vi "Parse Chat Reply from JSON.vi"(10 "stream":bool, 11 "Response JSON":string) -> (0 "openrouter reasoning":string, 1 "complete?":bool, 2 "message":T1, 3 "answer":string)   [LabVIEW 2023, in "LabVIEW LLM.lvlib"]
uses:
  LabVIEW LLM.lvlib
  chat-role.ctl
  chat-completion stream response.ctl
  chat-completion non-stream response.ctl
  openai_message.ctl
  <vilib>/addons/_JKI.lib/Serialization/JSON/JKI JSON Serialization.lvlib
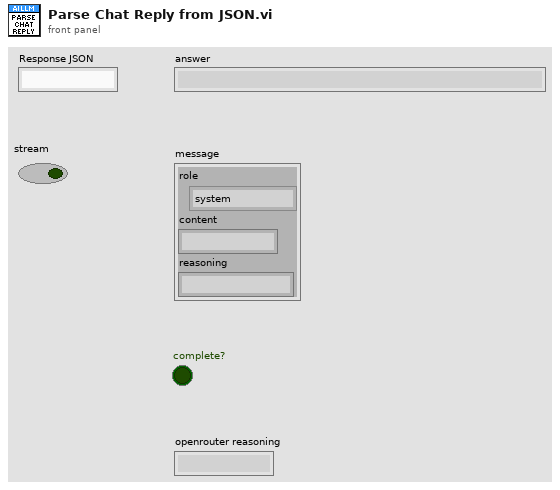
[diagram p1: front panel]
types:
  T1 = typedef "LabVIEW LLM.lvlib/openai_message.ctl" = cluster{"role":T2, "content":string, "reasoning":string}
  T2 = typedef "LabVIEW LLM.lvlib/chat-role.ctl" = enum16{"system", "user", "assistant"}
  T3 = typedef "LabVIEW LLM.lvlib/chat-completion stream response.ctl" = cluster{"id":string, "object":string, "created":i64, "model":string, "choices":cluster{"index":i64, "finish_reason":string, "delta":T1}[]}
  T4 = cluster{"index":i64, "finish_reason":string, "delta":T1}[]
  T5 = cluster{"index":i64, "finish_reason":string, "delta":T1}
  T6 = typedef "LabVIEW LLM.lvlib/chat-completion non-stream response.ctl" = cluster{"id":string, "object":string, "created":i64, "model":string, "choices":cluster{"index":i64, "finish_reason":string, "message":T1}[]}
  T7 = cluster{"index":i64, "finish_reason":string, "message":T1}[]
  T8 = cluster{"index":i64, "finish_reason":string, "message":T1}
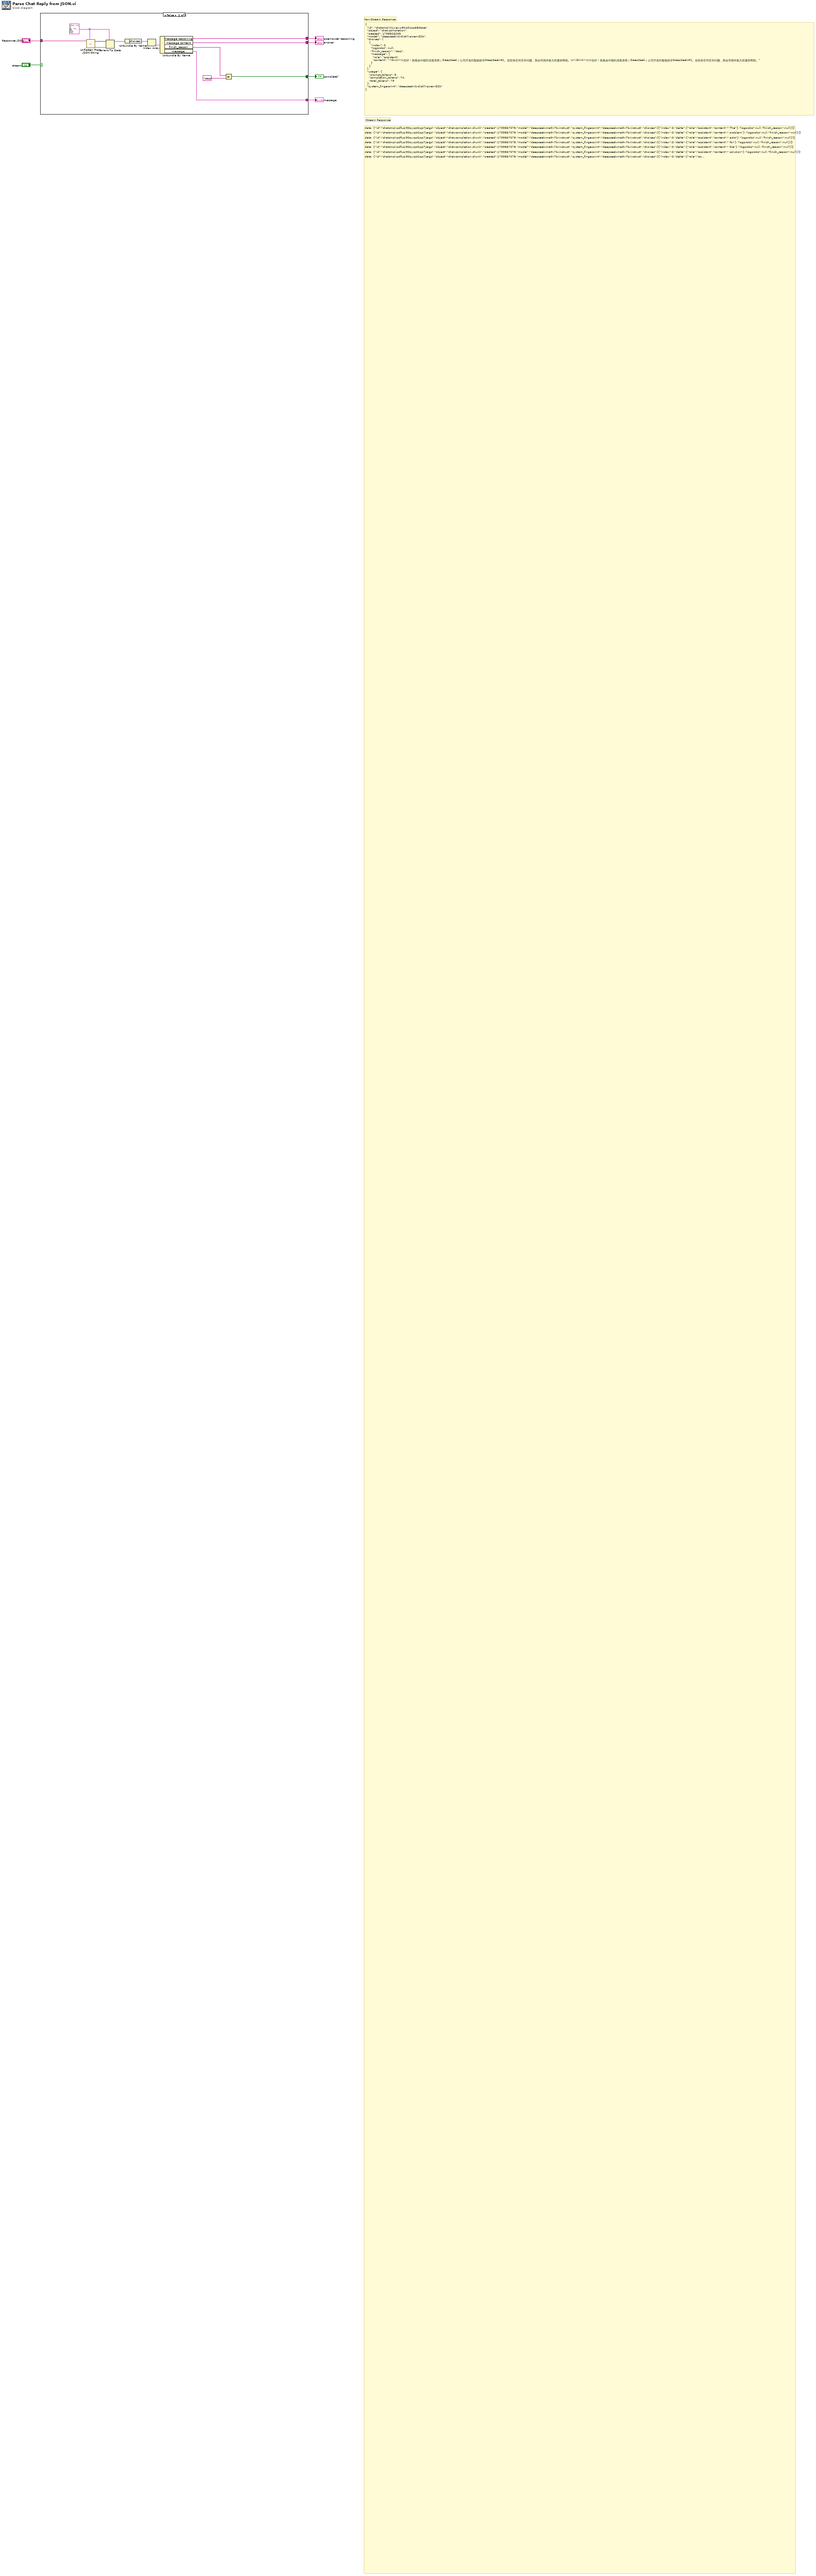
[diagram p0: block diagram]
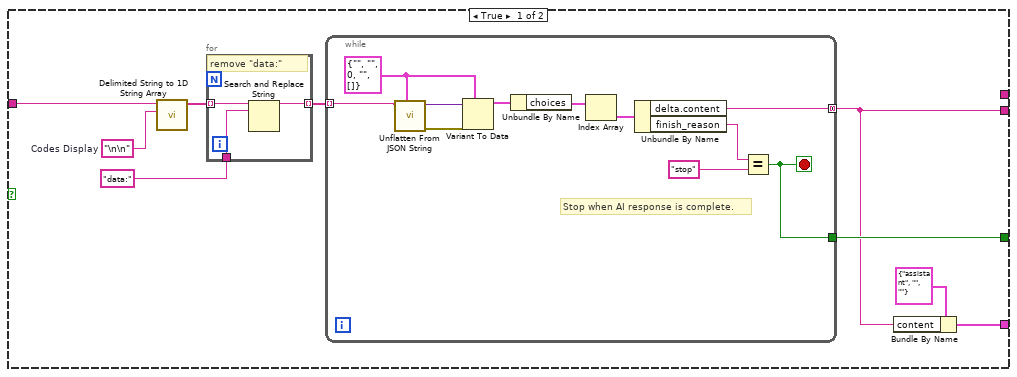
[diagram p2: hidden frame]
diagram:
  # "Non-Stream Response"
  # "Stream Response"
  # "data: {\"id\":\"chatcmpl-pdfuqi90oyqot1qp7jergc\",\"object\":\"chat.completion.chunk\",\"created\":1739867078,\"model\":\"deepseek-math-7b-instruct\",\"system_fingerprint\":\"deepseek-math-7b-instruct\",\"choices\":[{\"index\":0,\"delta\":{\"role\":\"assistant\",\"content\":\" The\"},\"logprobs\":null,\"finish_reason\":null}]}\n\ndata: {\"id\":\"chatcmpl-pdfuqi90oyqot1qp7jergc\",\"object\":\"chat.completion.chunk\",\"created\":1739867078,\"model\":\"deepseek-math-7b-instruct\",\"system_fingerprint\":\"deepseek-math-7b-instruct\",\"choices\":[{\"index\":0,\"delta\":{\"role\":\"assistant\",\"content\":\" problem\"},\"logprobs\":null,\"finish_reason\":null}]}\n\ndata: {\"id\":\"chatcmpl-pdfuqi90oyqot1qp7jergc\",\"object\":\"chat.completion.chunk\",\"created\":1739867078,\"model\":\"deepseek-math-7b-instruct\",\"system_fingerprint\":\"deepseek-math-7b-instruct\",\"choices\":[{\"index\":0,\"delta\":{\"role\":\"assistant\",\"content\":\" asks\"},\"logprobs\":null,\"finish_reason\":null}]}\n\ndata: {\"id\":\"chatcmpl-pdfuqi90oyqot1qp7jergc\",\"object\":\"chat.completion.chunk\",\"created\":1739867078,\"model\":\"deepseek-math-7b-instruct\",\"system_fingerprint\":\"deepseek-math-7b-instruct\",\"choices\":[{\"index\":0,\"delta\":{\"role\":\"assistant\",\"content\":\" for\"},\"logprobs\":null,\"finish_reason\":null}]}\n\ndata: {\"id\":\"chatcmpl-pdfuqi90oyqot1qp7jergc\",\"object\":\"chat.completion.chunk\",\"created\":1739867078,\"model\":\"deepseek-math-7b-instruct\",\"system_fingerprint\":\"deepseek-math-7b-instruct\",\"choices\":[{\"index\":0,\"delta\":{\"role\":\"assistant\",\"content\":\" the\"},\"logprobs\":null,\"finish_reason\":null}]}\n\ndata: {\"id\":\"chatcmpl-pdfuqi90oyqot1qp7jergc\",\"object\":\"chat.completion.chunk\",\"created\":1739867078,\"model\":\"deepseek-math-7b-instruct\",\"system_fingerprint\":\"deepseek-math-7b-instruct\",\"choices\":[{\"index\":0,\"delta\":{\"role\":\"assistant\",\"content\":\" solution\"},\"logprobs\":null,\"finish_reason\":null}]}\n\ndata: {\"id\":\"chatcmpl-pdfuqi90oyqot1qp7jergc\",\"object\":\"chat.completion.chunk\",\"created\":1739867078,\"model\":\"deepseek-math-7b-instruct\",\"system_fingerprint\":\"deepseek-math-7b-instruct\",\"choices\":[{\"index\":0,\"delta\":{\"role\":\"assistant\",\"content\":\" of\"},\"logprobs\":null,\"finish_reason\":null}]}\n\ndata: {\"id\":\"chatcmpl-pdfuqi90oyqot1qp7jergc\",\"object\":\"chat.completion.chunk\",\"created\":1739867078,\"model\":\"deepseek-math-7b-instruct\",\"system_fingerprint\":\"deepseek-math-7b-instruct\",\"choices\":[{\"index\":0,\"delta\":{\"role\":\"assistant\",\"content\":\"\\n\"},\"logprobs\":null,\"finish_reason\":null}]}\n\ndata: {\"id\":\"chatcmpl-pdfuqi90oyqot1qp7jergc\",\"object\":\"chat.completion.chunk\",\"created\":1739867078,\"model\":\"deepseek-math-7b-instruct\",\"system_fingerprint\":\"deepseek-math-7b-instruct\",\"choices\":[{\"index\":0,\"delta\":{\"role\":\"assistant\",\"content\":\"\\\\[\\\\\"},\"logprobs\":null,\"finish_reason\":null}]}\n\ndata: {\"id\":\"chatcmpl-pdfuqi90oyqot1qp7jergc\",\"object\":\"chat.completion.chunk\",\"created\":1739867078,\"model\":\"deepseek-math-7b-instruct\",\"system_fingerprint\":\"deepseek-math-7b-instruct\",\"choices\":[{\"index\":0,\"delta\":{\"role\":\"assistant\",\"content\":\"sin\"},\"logprobs\":null,\"finish_reason\":null}]}\n\ndata: {\"id\":\"chatcmpl-pdfuqi90oyqot1qp7jergc\",\"object\":\"chat.completion.chunk\",\"created\":1739867078,\"model\":\"deepseek-math-7b-instruct\",\"system_fingerprint\":\"deepseek-math-7b-instruct\",\"choices\":[{\"index\":0,\"delta\":{\"role\":\"assistant\",\"content\":\" x\"},\"logprobs\":null,\"finish_reason\":null}]}\n\ndata: {\"id\":\"chatcmpl-pdfuqi90oyqot1qp7jergc\",\"object\":\"chat.completion.chunk\",\"created\":1739867078,\"model\":\"deepseek-math-7b-instruct\",\"system_fingerprint\":\"deepseek-math-7b-instruct\",\"choices\":[{\"index\":0,\"delta\":{\"role\":\"assistant\",\"content\":\" +\"},\"logprobs\":null,\"finish_reason\":null}]}\n\ndata: {\"id\":\"chatcmpl-pdfuqi90oyqot1qp7jergc\",\"object\":\"chat.completion.chunk\",\"created\":1739867078,\"model\":\"deepseek-math-7b-instruct\",\"system_fingerprint\":\"deepseek-math-7b-instruct\",\"choices\":[{\"index\":0,\"delta\":{\"role\":\"assistant\",\"content\":\" \\\\\"},\"logprobs\":null,\"finish_reason\":null}]}\n\ndata: {\"id\":\"chatcmpl-pdfuqi90oyqot1qp7jergc\",\"object\":\"chat.completion.chunk\",\"created\":1739867078,\"model\":\"deepseek-math-7b-instruct\",\"system_fingerprint\":\"deepseek-math-7b-instruct\",\"choices\":[{\"index\":0,\"delta\":{\"role\":\"assistant\",\"content\":\"cos\"},\"logprobs\":null,\"finish_reason\":null}]}\n\ndata: {\"id\":\"chatcmpl-pdfuqi90oyqot1qp7jergc\",\"object\":\"chat.completion.chunk\",\"created\":1739867078,\"model\":\"deepseek-math-7b-instruct\",\"system_fingerprint\":\"deepseek-math-7b-instruct\",\"choices\":[{\"index\":0,\"delta\":{\"role\":\"assistant\",\"content\":\" \"},\"logprobs\":null,\"finish_reason\":null}]}\n\ndata: {\"id\":\"chatcmpl-pdfuqi90oyqot1qp7jergc\",\"object\":\"chat.completion.chunk\",\"created\":1739867078,\"model\":\"deepseek-math-7b-instruct\",\"system_fingerprint\":\"deepseek-math-7b-instruct\",\"choices\":[{\"index\":0,\"delta\":{\"role\":\"assistant\",\"content\":\"2\"},\"logprobs\":null,\"finish_reason\":null}]}\n\ndata: {\"id\":\"chatcmpl-pdfuqi90oyqot1qp7jergc\",\"object\":\"chat.completion.chunk\",\"created\":1739867078,\"model\":\"deepseek-math-7b-instruct\",\"system_fingerprint\":\"deepseek-math-7b-instruct\",\"choices\":[{\"index\":0,\"delta\":{\"role\":\"assistant\",\"content\":\"x\"},\"logprobs\":null,\"finish_reason\":null}]}\n\ndata: {\"id\":\"chatcmpl-pdfuqi90oyqot1qp7jergc\",\"object\":\"chat.completion.chunk\",\"created\":1739867078,\"model\":\"deepseek-math-7b-instruct\",\"system_fingerprint\":\"deepseek-math-7b-instruct\",\"choices\":[{\"index\":0,\"delta\":{\"role\":\"assistant\",\"content\":\" =\"},\"logprobs\":null,\"finish_reason\":null}]}\n\ndata: {\"id\":\"chatcmpl-pdfuqi90oyqot1qp7jergc\",\"object\":\"chat.completion.chunk\",\"created\":1739867078,\"model\":\"deepseek-math-7b-instruct\",\"system_fingerprint\":\"deepseek-math-7b-instruct\",\"choices\":[{\"index\":0,\"delta\":{\"role\":\"assistant\",\"content\":\" -\"},\"logprobs\":null,\"finish_reason\":null}]}\n\ndata: {\"id\":\"chatcmpl-pdfuqi90oyqot1qp7jergc\",\"object\":\"chat.completion.chunk\",\"created\":1739867078,\"model\":\"deepseek-math-7b-instruct\",\"system_fingerprint\":\"deepseek-math-7b-instruct\",\"choices\":[{\"index\":0,\"delta\":{\"role\":\"assistant\",\"content\":\"1\"},\"logprobs\":null,\"finish_reason\":null}]}\n\ndata: {\"id\":\"chatcmpl-pdfuqi90oyqot1qp7jergc\",\"object\":\"chat.completion.chunk\",\"created\":1739867078,\"model\":\"deepseek-math-7b-instruct\",\"system_fingerprint\":\"deepseek-math-7b-instruct\",\"choices\":[{\"index\":0,\"delta\":{\"role\":\"assistant\",\"content\":\".\\\\]\"},\"logprobs\":null,\"finish_reason\":null}]}\n\ndata: {\"id\":\"chatcmpl-pdfuqi90oyqot1qp7jergc\",\"object\":\"chat.completion.chunk\",\"created\":1739867078,\"model\":\"deepseek-math-7b-instruct\",\"system_fingerprint\":\"deepseek-math-7b-instruct\",\"choices\":[{\"index\":0,\"delta\":{\"role\":\"assistant\",\"content\":\"We\"},\"logprobs\":null,\"finish_reason\":null}]}\n\ndata: {\"id\":\"chatcmpl-pdfuqi90oyqot1qp7jergc\",\"object\":\"chat.completion.chunk\",\"created\":1739867078,\"model\":\"deepseek-math-7b-instruct\",\"system_fingerprint\":\"deepseek-math-7b-instruct\",\"choices\":[{\"index\":0,\"delta\":{\"role\":\"assistant\",\"content\":\" can\"},\"logprobs\":null,\"finish_reason\":null}]}\n\ndata: {\"id\":\"chatcmpl-pdfuqi90oyqot1qp7jergc\",\"object\":\"chat.completion.chunk\",\"created\":1739867078,\"model\":\"deepseek-math-7b-instruct\",\"system_fingerprint\":\"deepseek-math-7b-instruct\",\"choices\":[{\"index\":0,\"delta\":{\"role\":\"assistant\",\"content\":\" write\"},\"logprobs\":null,\"finish_reason\":null}]}\n\ndata: {\"id\":\"chatcmpl-pdfuqi90oyqot1qp7jergc\",\"object\":\"chat.completion.chunk\",\"created\":1739867078,\"model\":\"deepseek-math-7b-instruct\",\"system_fingerprint\":\"deepseek-math-7b-instruct\",\"choices\":[{\"index\":0,\"delta\":{\"role\":\"assistant\",\"content\":\" $\\\\\"},\"logprobs\":null,\"finish_reason\":null}]}\n\ndata: {\"id\":\"chatcmpl-pdfuqi90oyqot1qp7jergc\",\"object\":\"chat.completion.chunk\",\"created\":1739867078,\"model\":\"deepseek-math-7b-instruct\",\"system_fingerprint\":\"deepseek-math-7b-instruct\",\"choices\":[{\"index\":0,\"delta\":{\"role\":\"assistant\",\"content\":\"cos\"},\"logprobs\":null,\"finish_reason\":null}]}\n\ndata: {\"id\":\"chatcmpl-pdfuqi90oyqot1qp7jergc\",\"object\":\"chat.completion.chunk\",\"created\":1739867078,\"model\":\"deepseek-math-7b-instruct\",\"system_fingerprint\":\"deepseek-math-7b-instruct\",\"choices\":[{\"index\":0,\"delta\":{\"role\":\"assistant\",\"content\":\" \"},\"logprobs\":null,\"finish_reason\":null}]}\n\ndata: {\"id\":\"chatcmpl-pdfuqi90oyqot1qp7jergc\",\"object\":\"chat.completion.chunk\",\"created\":1739867078,\"model\":\"deepseek-math-7b-instruct\",\"system_fingerprint\":\"deepseek-math-7b-instruct\",\"choices\":[{\"index\":0,\"delta\":{\"role\":\"assistant\",\"content\":\"2\"},\"logprobs\":null,\"finish_reason\":null}]}\n\ndata: {\"id\":\"chatcmpl-pdfuqi90oyqot1qp7jergc\",\"object\":\"chat.completion.chunk\",\"created\":1739867078,\"model\":\"deepseek-math-7b-instruct\",\"system_fingerprint\":\"deepseek-math-7b-instruct\",\"choices\":[{\"index\":0,\"delta\":{\"role\":\"assistant\",\"content\":\"x\"},\"logprobs\":null,\"finish_reason\":null}]}\n\ndata: {\"id\":\"chatcmpl-pdfuqi90oyqot1qp7jergc\",\"object\":\"chat.completion.chunk\",\"created\":1739867078,\"model\":\"deepseek-math-7b-instruct\",\"system_fingerprint\":\"deepseek-math-7b-instruct\",\"choices\":[{\"index\":0,\"delta\":{\"role\":\"assistant\",\"content\":\"$\"},\"logprobs\":null,\"finish_reason\":null}]}\n\ndata: {\"id\":\"chatcmpl-pdfuqi90oyqot1qp7jergc\",\"object\":\"chat.completion.chunk\",\"created\":1739867078,\"model\":\"deepseek-math-7b-instruct\",\"system_fingerprint\":\"deepseek-math-7b-instruct\",\"choices\":[{\"index\":0,\"delta\":{\"role\":\"assistant\",\"content\":\" as\"},\"logprobs\":null,\"finish_reason\":null}]}\n\ndata: {\"id\":\"chatcmpl-pdfuqi90oyqot1qp7jergc\",\"object\":\"chat.completion.chunk\",\"created\":1739867078,\"model\":\"deepseek-math-7b-instruct\",\"system_fingerprint\":\"deepseek-math-7b-instruct\",\"choices\":[{\"index\":0,\"delta\":{\"role\":\"assistant\",\"content\":\" $\"},\"logprobs\":null,\"finish_reason\":null}]}\n\ndata: {\"id\":\"chatcmpl-pdfuqi90oyqot1qp7jergc\",\"object\":\"chat.completion.chunk\",\"created\":1739867078,\"model\":\"deepseek-math-7b-instruct\",\"system_fingerprint\":\"deepseek-math-7b-instruct\",\"choices\":[{\"index\":0,\"delta\":{\"role\":\"assistant\",\"content\":\"1\"},\"logprobs\":null,\"finish_reason\":null}]}\n\ndata: {\"id\":\"chatcmpl-pdfuqi90oyqot1qp7jergc\",\"object\":\"chat.completion.chunk\",\"created\":1739867078,\"model\":\"deepseek-math-7b-instruct\",\"system_fingerprint\":\"deepseek-math-7b-instruct\",\"choices\":[{\"index\":0,\"delta\":{\"role\":\"assistant\",\"content\":\"-\"},\"logprobs\":null,\"finish_reason\":null}]}\n\ndata: {\"id\":\"chatcmpl-pdfuqi90oyqot1qp7jergc\",\"object\":\"chat.completion.chunk\",\"created\":1739867078,\"model\":\"deepseek-math-7b-instruct\",\"system_fingerprint\":\"deepseek-math-7b-instruct\",\"choices\":[{\"index\":0,\"delta\":{\"role\":\"assistant\",\"content\":\"2\"},\"logprobs\":null,\"finish_reason\":null}]}\n\ndata: {\"id\":\"chatcmpl-pdfuqi90oyqot1qp7jergc\",\"object\":\"chat.completion.chunk\",\"created\":1739867078,\"model\":\"deepseek-math-7b-instruct\",\"system_fingerprint\":\"deepseek-math-7b-instruct\",\"choices\":[{\"index\":0,\"delta\":{\"role\":\"assistant\",\"content\":\"\\\\\"},\"logprobs\":null,\"finish_reason\":null}]}\n\ndata: {\"id\":\"chatcmpl-pdfuqi90oyqot1qp7jergc\",\"object\":\"chat.completion.chunk\",\"created\":1739867078,\"model\":\"deepseek-math-7b-instruct\",\"system_fingerprint\":\"deepseek-math-7b-instruct\",\"choices\":[{\"index\":0,\"delta\":{\"role\":\"assistant\",\"content\":\"sin\"},\"logprobs\":null,\"finish_reason\":null}]}\n\ndata: {\"id\":\"chatcmpl-pdfuqi90oyqot1qp7jergc\",\"object\":\"chat.completion.chunk\",\"created\":1739867078,\"model\":\"deepseek-math-7b-instruct\",\"system_fingerprint\":\"deepseek-math-7b-instruct\",\"choices\":[{\"index\":0,\"delta\":{\"role\":\"assistant\",\"content\":\"^\"},\"logprobs\":null,\"finish_reason\":null}]}\n\ndata: {\"id\":\"chatcmpl-pdfuqi90oyqot1qp7jergc\",\"object\":\"chat.completion.chunk\",\"created\":1739867078,\"model\":\"deepseek-math-7b-instruct\",\"system_fingerprint\":\"deepseek-math-7b-instruct\",\"choices\":[{\"index\":0,\"delta\":{\"role\":\"assistant\",\"content\":\"2\"},\"logprobs\":null,\"finish_reason\":null}]}\n\ndata: {\"id\":\"chatcmpl-pdfuqi90oyqot1qp7jergc\",\"object\":\"chat.completion.chunk\",\"created\":1739867078,\"model\":\"deepseek-math-7b-instruct\",\"system_fingerprint\":\"deepseek-math-7b-instruct\",\"choices\":[{\"index\":0,\"delta\":{\"role\":\"assistant\",\"content\":\" x\"},\"logprobs\":null,\"finish_reason\":null}]}\n\ndata: {\"id\":\"chatcmpl-pdfuqi90oyqot1qp7jergc\",\"object\":\"chat.completion.chunk\",\"created\":1739867078,\"model\":\"deepseek-math-7b-instruct\",\"system_fingerprint\":\"deepseek-math-7b-instruct\",\"choices\":[{\"index\":0,\"delta\":{\"role\":\"assistant\",\"content\":\"$,\"},\"logprobs\":null,\"finish_reason\":null}]}\n\ndata: {\"id\":\"chatcmpl-pdfuqi90oyqot1qp7jergc\",\"object\":\"chat.completion.chunk\",\"created\":1739867078,\"model\":\"deepseek-math-7b-instruct\",\"system_fingerprint\":\"deepseek-math-7b-instruct\",\"choices\":[{\"index\":0,\"delta\":{\"role\":\"assistant\",\"content\":\" so\"},\"logprobs\":null,\"finish_reason\":null}]}\n\ndata: {\"id\":\"chatcmpl-pdfuqi90oyqot1qp7jergc\",\"object\":\"chat.completion.chunk\",\"created\":1739867078,\"model\":\"deepseek-math-7b-instruct\",\"system_fingerprint\":\"deepseek-math-7b-instruct\",\"choices\":[{\"index\":0,\"delta\":{\"role\":\"assistant\",\"content\":\" we\"},\"logprobs\":null,\"finish_reason\":null}]}\n\ndata: {\"id\":\"chatcmpl-pdfuqi90oyqot1qp7jergc\",\"object\":\"chat.completion.chunk\",\"created\":1739867078,\"model\":\"deepseek-math-7b-instruct\",\"system_fingerprint\":\"deepseek-math-7b-instruct\",\"choices\":[{\"index\":0,\"delta\":{\"role\":\"assistant\",\"content\":\" have\"},\"logprobs\":null,\"finish_reason\":null}]}\n\ndata: {\"id\":\"chatcmpl-pdfuqi90oyqot1qp7jergc\",\"object\":\"chat.completion.chunk\",\"created\":1739867078,\"model\":\"deepseek-math-7b-instruct\",\"system_fingerprint\":\"deepseek-math-7b-instruct\",\"choices\":[{\"index\":0,\"delta\":{\"role\":\"assistant\",\"content\":\" \\\\[\\\\\"},\"logprobs\":null,\"finish_reason\":null}]}\n\ndata: {\"id\":\"chatcmpl-pdfuqi90oyqot1qp7jergc\",\"object\":\"chat.completion.chunk\",\"created\":1739867078,\"model\":\"deepseek-math-7b-instruct\",\"system_fingerprint\":\"deepseek-math-7b-instruct\",\"choices\":[{\"index\":0,\"delta\":{\"role\":\"assistant\",\"content\":\"sin\"},\"logprobs\":null,\"finish_reason\":null}]}\n\ndata: {\"id\":\"chatcmpl-pdfuqi90oyqot1qp7jergc\",\"object\":\"chat.completion.chunk\",\"created\":1739867078,\"model\":\"deepseek-math-7b-instruct\",\"system_fingerprint\":\"deepseek-math-7b-instruct\",\"choices\":[{\"index\":0,\"delta\":{\"role\":\"assistant\",\"content\":\" x\"},\"logprobs\":null,\"finish_reason\":null}]}\n\ndata: {\"id\":\"chatcmpl-pdfuqi90oyqot1qp7jergc\",\"object\":\"chat.completion.chunk\",\"created\":1739867078,\"model\":\"deepseek-math-7b-instruct\",\"system_fingerprint\":\"deepseek-math-7b-instruct\",\"choices\":[{\"index\":0,\"delta\":{\"role\":\"assistant\",\"content\":\" +\"},\"logprobs\":null,\"finish_reason\":null}]}\n\ndata: {\"id\":\"chatcmpl-pdfuqi90oyqot1qp7jergc\",\"object\":\"chat.completion.chunk\",\"created\":1739867078,\"model\":\"deepseek-math-7b-instruct\",\"system_fingerprint\":\"deepseek-math-7b-instruct\",\"choices\":[{\"index\":0,\"delta\":{\"role\":\"assistant\",\"content\":\" (\"},\"logprobs\":null,\"finish_reason\":null}]}\n\ndata: {\"id\":\"chatcmpl-pdfuqi90oyqot1qp7jergc\",\"object\":\"chat.completion.chunk\",\"created\":1739867078,\"model\":\"deepseek-math-7b-instruct\",\"system_fingerprint\":\"deepseek-math-7b-instruct\",\"choices\":[{\"index\":0,\"delta\":{\"role\":\"assistant\",\"content\":\"1\"},\"logprobs\":null,\"finish_reason\":null}]}\n\ndata: {\"id\":\"chatcmpl-pdfuqi90oyqot1qp7jergc\",\"object\":\"chat.completion.chunk\",\"created\":1739867078,\"model\":\"deepseek-math-7b-instruct\",\"system_fingerprint\":\"deepseek-math-7b-instruct\",\"choices\":[{\"index\":0,\"delta\":{\"role\":\"assistant\",\"content\":\" -\"},\"logprobs\":null,\"finish_reason\":null}]}\n\ndata: {\"id\":\"chatcmpl-pdfuqi90oyqot1qp7jergc\",\"object\":\"chat.completion.chunk\",\"created\":1739867078,\"model\":\"deepseek-math-7b-instruct\",\"system_fingerprint\":\"deepseek-math-7b-instruct\",\"choices\":[{\"index\":0,\"delta\":{\"role\":\"assistant\",\"content\":\" \"},\"logprobs\":null,\"finish_reason\":null}]}\n\ndata: {\"id\":\"chatcmpl-pdfuqi90oyqot1qp7jergc\",\"object\":\"chat.completion.chunk\",\"created\":1739867078,\"model\":\"deepseek-math-7b-instruct\",\"system_fingerprint\":\"deepseek-math-7b-instruct\",\"choices\":[{\"index\":0,\"delta\":{\"role\":\"assistant\",\"content\":\"2\"},\"logprobs\":null,\"finish_reason\":null}]}\n\ndata: {\"id\":\"chatcmpl-pdfuqi90oyqot1qp7jergc\",\"object\":\"chat.completion.chunk\",\"created\":1739867078,\"model\":\"deepseek-math-7b-instruct\",\"system_fingerprint\":\"deepseek-math-7b-instruct\",\"choices\":[{\"index\":0,\"delta\":{\"role\":\"assistant\",\"content\":\"\\\\\"},\"logprobs\":null,\"finish_reason\":null}]}\n\ndata: {\"id\":\"chatcmpl-pdfuqi90oyqot1qp7jergc\",\"object\":\"chat.completion.chunk\",\"created\":1739867078,\"model\":\"deepseek-math-7b-instruct\",\"system_fingerprint\":\"deepseek-math-7b-instruct\",\"choices\":[{\"index\":0,\"delta\":{\"role\":\"assistant\",\"content\":\"sin\"},\"logprobs\":null,\"finish_reason\":null}]}\n\ndata: {\"id\":\"chatcmpl-pdfuqi90oyqot1qp7jergc\",\"object\":\"chat.completion.chunk\",\"created\":1739867078,\"model\":\"deepseek-math-7b-instruct\",\"system_fingerprint\":\"deepseek-math-7b-instruct\",\"choices\":[{\"index\":0,\"delta\":{\"role\":\"assistant\",\"content\":\"^\"},\"logprobs\":null,\"finish_reason\":null}]}\n\ndata: {\"id\":\"chatcmpl-pdfuqi90oyqot1qp7jergc\",\"object\":\"chat.completion.chunk\",\"created\":1739867078,\"model\":\"deepseek-math-7b-instruct\",\"system_fingerprint\":\"deepseek-math-7b-instruct\",\"choices\":[{\"index\":0,\"delta\":{\"role\":\"assistant\",\"content\":\"2\"},\"logprobs\":null,\"finish_reason\":null}]}\n\ndata: {\"id\":\"chatcmpl-pdfuqi90oyqot1qp7jergc\",\"object\":\"chat.completion.chunk\",\"created\":1739867078,\"model\":\"deepseek-math-7b-instruct\",\"system_fingerprint\":\"deepseek-math-7b-instruct\",\"choices\":[{\"index\":0,\"delta\":{\"role\":\"assistant\",\"content\":\" x\"},\"logprobs\":null,\"finish_reason\":null}]}\n\ndata: {\"id\":\"chatcmpl-pdfuqi90oyqot1qp7jergc\",\"object\":\"chat.completion.chunk\",\"created\":1739867078,\"model\":\"deepseek-math-7b-instruct\",\"system_fingerprint\":\"deepseek-math-7b-instruct\",\"choices\":[{\"index\":0,\"delta\":{\"role\":\"assistant\",\"content\":\")\"},\"logprobs\":null,\"finish_reason\":null}]}\n\ndata: {\"id\":\"chatcmpl-pdfuqi90oyqot1qp7jergc\",\"object\":\"chat.completion.chunk\",\"created\":1739867078,\"model\":\"deepseek-math-7b-instruct\",\"system_fingerprint\":\"deepseek-math-7b-instruct\",\"choices\":[{\"index\":0,\"delta\":{\"role\":\"assistant\",\"content\":\" =\"},\"logprobs\":null,\"finish_reason\":null}]}\n\ndata: {\"id\":\"chatcmpl-pdfuqi90oyqot1qp7jergc\",\"object\":\"chat.completion.chunk\",\"created\":1739867078,\"model\":\"deepseek-math-7b-instruct\",\"system_fingerprint\":\"deepseek-math-7b-instruct\",\"choices\":[{\"index\":0,\"delta\":{\"role\":\"assistant\",\"content\":\" -\"},\"logprobs\":null,\"finish_reason\":null}]}\n\ndata: {\"id\":\"chatcmpl-pdfuqi90oyqot1qp7jergc\",\"object\":\"chat.completion.chunk\",\"created\":1739867078,\"model\":\"deepseek-math-7b-instruct\",\"system_fingerprint\":\"deepseek-math-7b-instruct\",\"choices\":[{\"index\":0,\"delta\":{\"role\":\"assistant\",\"content\":\"1\"},\"logprobs\":null,\"finish_reason\":null}]}\n\ndata: {\"id\":\"chatcmpl-pdfuqi90oyqot1qp7jergc\",\"object\":\"chat.completion.chunk\",\"created\":1739867078,\"model\":\"deepseek-math-7b-instruct\",\"system_fingerprint\":\"deepseek-math-7b-instruct\",\"choices\":[{\"index\":0,\"delta\":{\"role\":\"assistant\",\"content\":\",\\\\]\"},\"logprobs\":null,\"finish_reason\":null}]}\n\ndata: {\"id\":\"chatcmpl-pdfuqi90oyqot1qp7jergc\",\"object\":\"chat.completion.chunk\",\"created\":1739867078,\"model\":\"deepseek-math-7b-instruct\",\"system_fingerprint\":\"deepseek-math-7b-instruct\",\"choices\":[{\"index\":0,\"delta\":{\"role\":\"assistant\",\"content\":\"which\"},\"logprobs\":null,\"finish_reason\":null}]}\n\ndata: {\"id\":\"chatcmpl-pdfuqi90oyqot1qp7jergc\",\"object\":\"chat.completion.chunk\",\"created\":1739867078,\"model\":\"deepseek-math-7b-instruct\",\"system_fingerprint\":\"deepseek-math-7b-instruct\",\"choices\":[{\"index\":0,\"delta\":{\"role\":\"assistant\",\"content\":\" simplifies\"},\"logprobs\":null,\"finish_reason\":null}]}\n\ndata: {\"id\":\"chatcmpl-pdfuqi90oyqot1qp7jergc\",\"object\":\"chat.completion.chunk\",\"created\":1739867078,\"model\":\"deepseek-math-7b-instruct\",\"system_fingerprint\":\"deepseek-math-7b-instruct\",\"choices\":[{\"index\":0,\"delta\":{\"role\":\"assistant\",\"content\":\" to\"},\"logprobs\":null,\"finish_reason\":null}]}\n\ndata: {\"id\":\"chatcmpl-pdfuqi90oyqot1qp7jergc\",\"object\":\"chat.completion.chunk\",\"created\":1739867078,\"model\":\"deepseek-math-7b-instruct\",\"system_fingerprint\":\"deepseek-math-7b-instruct\",\"choices\":[{\"index\":0,\"delta\":{\"role\":\"assistant\",\"content\":\" \\\\[\"},\"logprobs\":null,\"finish_reason\":null}]}\n\ndata: {\"id\":\"chatcmpl-pdfuqi90oyqot1qp7jergc\",\"object\":\"chat.completion.chunk\",\"created\":1739867078,\"model\":\"deepseek-math-7b-instruct\",\"system_fingerprint\":\"deepseek-math-7b-instruct\",\"choices\":[{\"index\":0,\"delta\":{\"role\":\"assistant\",\"content\":\"0\"},\"logprobs\":null,\"finish_reason\":null}]}\n\ndata: {\"id\":\"chatcmpl-pdfuqi90oyqot1qp7jergc\",\"object\":\"chat.completion.chunk\",\"created\":1739867078,\"model\":\"deepseek-math-7b-instruct\",\"system_fingerprint\":\"deepseek-math-7b-instruct\",\"choices\":[{\"index\":0,\"delta\":{\"role\":\"assistant\",\"content\":\"=\"},\"logprobs\":null,\"finish_reason\":null}]}\n\ndata: {\"id\":\"chatcmpl-pdfuqi90oyqot1qp7jergc\",\"object\":\"chat.completion.chunk\",\"created\":1739867078,\"model\":\"deepseek-math-7b-instruct\",\"system_fingerprint\":\"deepseek-math-7b-instruct\",\"choices\":[{\"index\":0,\"delta\":{\"role\":\"assistant\",\"content\":\"2\"},\"logprobs\":null,\"finish_reason\":null}]}\n\ndata: {\"id\":\"chatcmpl-pdfuqi90oyqot1qp7jergc\",\"object\":\"chat.completion.chunk\",\"created\":1739867078,\"model\":\"deepseek-math-7b-instruct\",\"system_fingerprint\":\"deepseek-math-7b-instruct\",\"choices\":[{\"index\":0,\"delta\":{\"role\":\"assistant\",\"content\":\"\\\\\"},\"logprobs\":null,\"finish_reason\":null}]}\n\ndata: {\"id\":\"chatcmpl-pdfuqi90oyqot1qp7jergc\",\"object\":\"chat.completion.chunk\",\"created\":1739867078,\"model\":\"deepseek-math-7b-instruct\",\"system_fingerprint\":\"deepseek-math-7b-instruct\",\"choices\":[{\"index\":0,\"delta\":{\"role\":\"assistant\",\"content\":\"sin\"},\"logprobs\":null,\"finish_reason\":null}]}\n\ndata: {\"id\":\"chatcmpl-pdfuqi90oyqot1qp7jergc\",\"object\":\"chat.completion.chunk\",\"created\":1739867078,\"model\":\"deepseek-math-7b-instruct\",\"system_fingerprint\":\"deepseek-math-7b-instruct\",\"choices\":[{\"index\":0,\"delta\":{\"role\":\"assistant\",\"content\":\" ^\"},\"logprobs\":null,\"finish_reason\":null}]}\n\ndata: {\"id\":\"chatcmpl-pdfuqi90oyqot1qp7jergc\",\"object\":\"chat.completion.chunk\",\"created\":1739867078,\"model\":\"deepseek-math-7b-instruct\",\"system_fingerprint\":\"deepseek-math-7b-instruct\",\"choices\":[{\"index\":0,\"delta\":{\"role\":\"assistant\",\"content\":\"2\"},\"logprobs\":null,\"finish_reason\":null}]}\n\ndata: {\"id\":\"chatcmpl-pdfuqi90oyqot1qp7jergc\",\"object\":\"chat.completion.chunk\",\"created\":1739867078,\"model\":\"deepseek-math-7b-instruct\",\"system_fingerprint\":\"deepseek-math-7b-instruct\",\"choices\":[{\"index\":0,\"delta\":{\"role\":\"assistant\",\"content\":\"(\"},\"logprobs\":null,\"finish_reason\":null}]}\n\ndata: {\"id\":\"chatcmpl-pdfuqi90oyqot1qp7jergc\",\"object\":\"chat.completion.chunk\",\"created\":1739867078,\"model\":\"deepseek-math-7b-instruct\",\"system_fingerprint\":\"deepseek-math-7b-instruct\",\"choices\":[{\"index\":0,\"delta\":{\"role\":\"assistant\",\"content\":\"x\"},\"logprobs\":null,\"finish_reason\":null}]}\n\ndata: {\"id\":\"chatcmpl-pdfuqi90oyqot1qp7jergc\",\"object\":\"chat.completion.chunk\",\"created\":1739867078,\"model\":\"deepseek-math-7b-instruct\",\"system_fingerprint\":\"deepseek-math-7b-instruct\",\"choices\":[{\"index\":0,\"delta\":{\"role\":\"assistant\",\"content\":\")+\\\\\"},\"logprobs\":null,\"finish_reason\":null}]}\n\ndata: {\"id\":\"chatcmpl-pdfuqi90oyqot1qp7jergc\",\"object\":\"chat.completion.chunk\",\"created\":1739867078,\"model\":\"deepseek-math-7b-instruct\",\"system_fingerprint\":\"deepseek-math-7b-instruct\",\"choices\":[{\"index\":0,\"delta\":{\"role\":\"assistant\",\"content\":\"sin\"},\"logprobs\":null,\"finish_reason\":null}]}\n\ndata: {\"id\":\"chatcmpl-pdfuqi90oyqot1qp7jergc\",\"object\":\"chat.completion.chunk\",\"created\":1739867078,\"model\":\"deepseek-math-7b-instruct\",\"system_fingerprint\":\"deepseek-math-7b-instruct\",\"choices\":[{\"index\":0,\"delta\":{\"role\":\"assistant\",\"content\":\"(\"},\"logprobs\":null,\"finish_reason\":null}]}\n\ndata: {\"id\":\"chatcmpl-pdfuqi90oyqot1qp7jergc\",\"object\":\"chat.completion.chunk\",\"created\":1739867078,\"model\":\"deepseek-math-7b-instruct\",\"system_fingerprint\":\"deepseek-math-7b-instruct\",\"choices\":[{\"index\":0,\"delta\":{\"role\":\"assistant\",\"content\":\"x\"},\"logprobs\":null,\"finish_reason\":null}]}\n\ndata: {\"id\":\"chatcmpl-pdfuqi90oyqot1qp7jergc\",\"object\":\"chat.completion.chunk\",\"created\":1739867078,\"model\":\"deepseek-math-7b-instruct\",\"system_fingerprint\":\"deepseek-math-7b-instruct\",\"choices\":[{\"index\":0,\"delta\":{\"role\":\"assistant\",\"content\":\")+\"},\"logprobs\":null,\"finish_reason\":null}]}\n\ndata: {\"id\":\"chatcmpl-pdfuqi90oyqot1qp7jergc\",\"object\":\"chat.completion.chunk\",\"created\":1739867078,\"model\":\"deepseek-math-7b-instruct\",\"system_fingerprint\":\"deepseek-math-7b-instruct\",\"choices\":[{\"index\":0,\"delta\":{\"role\":\"assistant\",\"content\":\"1\"},\"logprobs\":null,\"finish_reason\":null}]}\n\ndata: {\"id\":\"chatcmpl-pdfuqi90oyqot1qp7jergc\",\"object\":\"chat.completion.chunk\",\"created\":1739867078,\"model\":\"deepseek-math-7b-instruct\",\"system_fingerprint\":\"deepseek-math-7b-instruct\",\"choices\":[{\"index\":0,\"delta\":{\"role\":\"assistant\",\"content\":\"\\\\]\"},\"logprobs\":null,\"finish_reason\":null}]}\n\ndata: {\"id\":\"chatcmpl-pdfuqi90oyqot1qp7jergc\",\"object\":\"chat.completion.chunk\",\"created\":1739867078,\"model\":\"deepseek-math-7b-instruct\",\"system_fingerprint\":\"deepseek-math-7b-instruct\",\"choices\":[{\"index\":0,\"delta\":{\"role\":\"assistant\",\"content\":\"or\"},\"logprobs\":null,\"finish_reason\":null}]}\n\ndata: {\"id\":\"chatcmpl-pdfuqi90oyqot1qp7jergc\",\"object\":\"chat.completion.chunk\",\"created\":1739867078,\"model\":\"deepseek-math-7b-instruct\",\"system_fingerprint\":\"deepseek-math-7b-instruct\",\"choices\":[{\"index\":0,\"delta\":{\"role\":\"assistant\",\"content\":\",\"},\"logprobs\":null,\"finish_reason\":null}]}\n\ndata: {\"id\":\"chatcmpl-pdfuqi90oyqot1qp7jergc\",\"object\":\"chat.completion.chunk\",\"created\":1739867078,\"model\":\"deepseek-math-7b-instruct\",\"system_fingerprint\":\"deepseek-math-7b-instruct\",\"choices\":[{\"index\":0,\"delta\":{\"role\":\"assistant\",\"content\":\" equivalently\"},\"logprobs\":null,\"finish_reason\":null}]}\n\ndata: {\"id\":\"chatcmpl-pdfuqi90oyqot1qp7jergc\",\"object\":\"chat.completion.chunk\",\"created\":1739867078,\"model\":\"deepseek-math-7b-instruct\",\"system_fingerprint\":\"deepseek-math-7b-instruct\",\"choices\":[{\"index\":0,\"delta\":{\"role\":\"assistant\",\"content\":\",\\\\\"},\"logprobs\":null,\"finish_reason\":null}]}\n\ndata: {\"id\":\"chatcmpl-pdfuqi90oyqot1qp7jergc\",\"object\":\"chat.completion.chunk\",\"created\":1739867078,\"model\":\"deepseek-math-7b-instruct\",\"system_fingerprint\":\"deepseek-math-7b-instruct\",\"choices\":[{\"index\":0,\"delta\":{\"role\":\"assistant\",\"content\":\"[\"},\"logprobs\":null,\"finish_reason\":null}]}\n\ndata: {\"id\":\"chatcmpl-pdfuqi90oyqot1qp7jergc\",\"object\":\"chat.completion.chunk\",\"created\":1739867078,\"model\":\"deepseek-math-7b-instruct\",\"system_fingerprint\":\"deepseek-math-7b-instruct\",\"choices\":[{\"index\":0,\"delta\":{\"role\":\"assistant\",\"content\":\"2\"},\"logprobs\":null,\"finish_reason\":null}]}\n\ndata: {\"id\":\"chatcmpl-pdfuqi90oyqot1qp7jergc\",\"object\":\"chat.completion.chunk\",\"created\":1739867078,\"model\":\"deepseek-math-7b-instruct\",\"system_fingerprint\":\"deepseek-math-7b-instruct\",\"choices\":[{\"index\":0,\"delta\":{\"role\":\"assistant\",\"content\":\" \\\\\"},\"logprobs\":null,\"finish_reason\":null}]}\n\ndata: {\"id\":\"chatcmpl-pdfuqi90oyqot1qp7jergc\",\"object\":\"chat.completion.chunk\",\"created\":1739867078,\"model\":\"deepseek-math-7b-instruct\",\"system_fingerprint\":\"deepseek-math-7b-instruct\",\"choices\":[{\"index\":0,\"delta\":{\"role\":\"assistant\",\"content\":\"sin\"},\"logprobs\":null,\"finish_reason\":null}]}\n\ndata: {\"id\":\"chatcmpl-pdfuqi90oyqot1qp7jergc\",\"object\":\"chat.completion.chunk\",\"created\":1739867078,\"model\":\"deepseek-math-7b-instruct\",\"system_fingerprint\":\"deepseek-math-7b-instruct\",\"choices\":[{\"index\":0,\"delta\":{\"role\":\"assistant\",\"content\":\"^\"},\"logprobs\":null,\"finish_reason\":null}]}\n\ndata: {\"id\":\"chatcmpl-pdfuqi90oyqot1qp7jergc\",\"object\":\"chat.completion.chunk\",\"created\":1739867078,\"model\":\"deepseek-math-7b-instruct\",\"system_fingerprint\":\"deepseek-math-7b-instruct\",\"choices\":[{\"index\":0,\"delta\":{\"role\":\"assistant\",\"content\":\"2\"},\"logprobs\":null,\"finish_reason\":null}]}\n\ndata: {\"id\":\"chatcmpl-pdfuqi90oyqot1qp7jergc\",\"object\":\"chat.completion.chunk\",\"created\":1739867078,\"model\":\"deepseek-math-7b-instruct\",\"system_fingerprint\":\"deepseek-math-7b-instruct\",\"choices\":[{\"index\":0,\"delta\":{\"role\":\"assistant\",\"content\":\" x\"},\"logprobs\":null,\"finish_reason\":null}]}\n\ndata: {\"id\":\"chatcmpl-pdfuqi90oyqot1qp7jergc\",\"object\":\"chat.completion.chunk\",\"created\":1739867078,\"model\":\"deepseek-math-7b-instruct\",\"system_fingerprint\":\"deepseek-math-7b-instruct\",\"choices\":[{\"index\":0,\"delta\":{\"role\":\"assistant\",\"content\":\"+\\\\\"},\"logprobs\":null,\"finish_reason\":null}]}\n\ndata: {\"id\":\"chatcmpl-pdfuqi90oyqot1qp7jergc\",\"object\":\"chat.completion.chunk\",\"created\":1739867078,\"model\":\"deepseek-math-7b-instruct\",\"system_fingerprint\":\"deepseek-math-7b-instruct\",\"choices\":[{\"index\":0,\"delta\":{\"role\":\"assistant\",\"content\":\"sin\"},\"logprobs\":null,\"finish_reason\":null}]}\n\ndata: {\"id\":\"chatcmpl-pdfuqi90oyqot1qp7jergc\",\"object\":\"chat.completion.chunk\",\"created\":1739867078,\"model\":\"deepseek-math-7b-instruct\",\"system_fingerprint\":\"deepseek-math-7b-instruct\",\"choices\":[{\"index\":0,\"delta\":{\"role\":\"assistant\",\"content\":\" x\"},\"logprobs\":null,\"finish_reason\":null}]}\n\ndata: {\"id\":\"chatcmpl-pdfuqi90oyqot1qp7jergc\",\"object\":\"chat.completion.chunk\",\"created\":1739867078,\"model\":\"deepseek-math-7b-instruct\",\"system_fingerprint\":\"deepseek-math-7b-instruct\",\"choices\":[{\"index\":0,\"delta\":{\"role\":\"assistant\",\"content\":\"+\"},\"logprobs\":null,\"finish_reason\":null}]}\n\ndata: {\"id\":\"chatcmpl-pdfuqi90oyqot1qp7jergc\",\"object\":\"chat.completion.chunk\",\"created\":1739867078,\"model\":\"deepseek-math-7b-instruct\",\"system_fingerprint\":\"deepseek-math-7b-instruct\",\"choices\":[{\"index\":0,\"delta\":{\"role\":\"assistant\",\"content\":\"1\"},\"logprobs\":null,\"finish_reason\":null}]}\n\ndata: {\"id\":\"chatcmpl-pdfuqi90oyqot1qp7jergc\",\"object\":\"chat.completion.chunk\",\"created\":1739867078,\"model\":\"deepseek-math-7b-instruct\",\"system_fingerprint\":\"deepseek-math-7b-instruct\",\"choices\":[{\"index\":0,\"delta\":{\"role\":\"assistant\",\"content\":\"=(\"},\"logprobs\":null,\"finish_reason\":null}]}\n\ndata: {\"id\":\"chatcmpl-pdfuqi90oyqot1qp7jergc\",\"object\":\"chat.completion.chunk\",\"created\":1739867078,\"model\":\"deepseek-math-7b-instruct\",\"system_fingerprint\":\"deepseek-math-7b-instruct\",\"choices\":[{\"index\":0,\"delta\":{\"role\":\"assistant\",\"content\":\"2\"},\"logprobs\":null,\"finish_reason\":null}]}\n\ndata: {\"id\":\"chatcmpl-pdfuqi90oyqot1qp7jergc\",\"object\":\"chat.completion.chunk\",\"created\":1739867078,\"model\":\"deepseek-math-7b-instruct\",\"system_fingerprint\":\"deepseek-math-7b-instruct\",\"choices\":[{\"index\":0,\"delta\":{\"role\":\"assistant\",\"content\":\" \\\\\"},\"logprobs\":null,\"finish_reason\":null}]}\n\ndata: {\"id\":\"chatcmpl-pdfuqi90oyqot1qp7jergc\",\"object\":\"chat.completion.chunk\",\"created\":1739867078,\"model\":\"deepseek-math-7b-instruct\",\"system_fingerprint\":\"deepseek-math-7b-instruct\",\"choices\":[{\"index\":0,\"delta\":{\"role\":\"assistant\",\"content\":\"sin\"},\"logprobs\":null,\"finish_reason\":null}]}\n\ndata: {\"id\":\"chatcmpl-pdfuqi90oyqot1qp7jergc\",\"object\":\"chat.completion.chunk\",\"created\":1739867078,\"model\":\"deepseek-math-7b-instruct\",\"system_fingerprint\":\"deepseek-math-7b-instruct\",\"choices\":[{\"index\":0,\"delta\":{\"role\":\"assistant\",\"content\":\" x\"},\"logprobs\":null,\"finish_reason\":null}]}\n\ndata: {\"id\":\"chatcmpl-pdfuqi90oyqot1qp7jergc\",\"object\":\"chat.completion.chunk\",\"created\":1739867078,\"model\":\"deepseek-math-7b-instruct\",\"system_fingerprint\":\"deepseek-math-7b-instruct\",\"choices\":[{\"index\":0,\"delta\":{\"role\":\"assistant\",\"content\":\"+\"},\"logprobs\":null,\"finish_reason\":null}]}\n\ndata: {\"id\":\"chatcmpl-pdfuqi90oyqot1qp7jergc\",\"object\":\"chat.completion.chunk\",\"created\":1739867078,\"model\":\"deepseek-math-7b-instruct\",\"system_fingerprint\":\"deepseek-math-7b-instruct\",\"choices\":[{\"index\":0,\"delta\":{\"role\":\"assistant\",\"content\":\"1\"},\"logprobs\":null,\"finish_reason\":null}]}\n\ndata: {\"id\":\"chatcmpl-pdfuqi90oyqot1qp7jergc\",\"object\":\"chat.completion.chunk\",\"created\":1739867078,\"model\":\"deepseek-math-7b-instruct\",\"system_fingerprint\":\"deepseek-math-7b-instruct\",\"choices\":[{\"index\":0,\"delta\":{\"role\":\"assistant\",\"content\":\")(\\\\\"},\"logprobs\":null,\"finish_reason\":null}]}\n\ndata: {\"id\":\"chatcmpl-pdfuqi90oyqot1qp7jergc\",\"object\":\"chat.completion.chunk\",\"created\":1739867078,\"model\":\"deepseek-math-7b-instruct\",\"system_fingerprint\":\"deepseek-math-7b-instruct\",\"choices\":[{\"index\":0,\"delta\":{\"role\":\"assistant\",\"content\":\"sin\"},\"logprobs\":null,\"finish_reason\":null}]}\n\ndata: {\"id\":\"chatcmpl-pdfuqi90oyqot1qp7jergc\",\"object\":\"chat.completion.chunk\",\"created\":1739867078,\"model\":\"deepseek-math-7b-instruct\",\"system_fingerprint\":\"deepseek-math-7b-instruct\",\"choices\":[{\"index\":0,\"delta\":{\"role\":\"assistant\",\"content\":\" x\"},\"logprobs\":null,\"finish_reason\":null}]}\n\ndata: {\"id\":\"chatcmpl-pdfuqi90oyqot1qp7jergc\",\"object\":\"chat.completion.chunk\",\"created\":1739867078,\"model\":\"deepseek-math-7b-instruct\",\"system_fingerprint\":\"deepseek-math-7b-instruct\",\"choices\":[{\"index\":0,\"delta\":{\"role\":\"assistant\",\"content\":\"+\"},\"logprobs\":null,\"finish_reason\":null}]}\n\ndata: {\"id\":\"chatcmpl-pdfuqi90oyqot1qp7jergc\",\"object\":\"chat.completion.chunk\",\"created\":1739867078,\"model\":\"deepseek-math-7b-instruct\",\"system_fingerprint\":\"deepseek-math-7b-instruct\",\"choices\":[{\"index\":0,\"delta\":{\"role\":\"assistant\",\"content\":\"1\"},\"logprobs\":null,\"finish_reason\":null}]}\n\ndata: {\"id\":\"chatcmpl-pdfuqi90oyqot1qp7jergc\",\"object\":\"chat.completion.chunk\",\"created\":1739867078,\"model\":\"deepseek-math-7b-instruct\",\"system_fingerprint\":\"deepseek-math-7b-instruct\",\"choices\":[{\"index\":0,\"delta\":{\"role\":\"assistant\",\"content\":\")=\"},\"logprobs\":null,\"finish_reason\":null}]}\n\ndata: {\"id\":\"chatcmpl-pdfuqi90oyqot1qp7jergc\",\"object\":\"chat.completion.chunk\",\"created\":1739867078,\"model\":\"deepseek-math-7b-instruct\",\"system_fingerprint\":\"deepseek-math-7b-instruct\",\"choices\":[{\"index\":0,\"delta\":{\"role\":\"assistant\",\"content\":\"0\"},\"logprobs\":null,\"finish_reason\":null}]}\n\ndata: {\"id\":\"chatcmpl-pdfuqi90oyqot1qp7jergc\",\"object\":\"chat.completion.chunk\",\"created\":1739867078,\"model\":\"deepseek-math-7b-instruct\",\"system_fingerprint\":\"deepseek-math-7b-instruct\",\"choices\":[{\"index\":0,\"delta\":{\"role\":\"assistant\",\"content\":\".\\\\]\"},\"logprobs\":null,\"finish_reason\":null}]}\n\ndata: {\"id\":\"chatcmpl-pdfuqi90oyqot1qp7jergc\",\"object\":\"chat.completion.chunk\",\"created\":1739867078,\"model\":\"deepseek-math-7b-instruct\",\"system_fingerprint\":\"deepseek-math-7b-instruct\",\"choices\":[{\"index\":0,\"delta\":{\"role\":\"assistant\",\"content\":\"Therefore\"},\"logprobs\":null,\"finish_reason\":null}]}\n\ndata: {\"id\":\"chatcmpl-pdfuqi90oyqot1qp7jergc\",\"object\":\"chat.completion.chunk\",\"created\":1739867078,\"model\":\"deepseek-math-7b-instruct\",\"system_fingerprint\":\"deepseek-math-7b-instruct\",\"choices\":[{\"index\":0,\"delta\":{\"role\":\"assistant\",\"content\":\" we\"},\"logprobs\":null,\"finish_reason\":null}]}\n\ndata: {\"id\":\"chatcmpl-pdfuqi90oyqot1qp7jergc\",\"object\":\"chat.completion.chunk\",\"created\":1739867078,\"model\":\"deepseek-math-7b-instruct\",\"system_fingerprint\":\"deepseek-math-7b-instruct\",\"choices\":[{\"index\":0,\"delta\":{\"role\":\"assistant\",\"content\":\" have\"},\"logprobs\":null,\"finish_reason\":null}]}\n\ndata: {\"id\":\"chatcmpl-pdfuqi90oyqot1qp7jergc\",\"object\":\"chat.completion.chunk\",\"created\":1739867078,\"model\":\"deepseek-math-7b-instruct\",\"system_fingerprint\":\"deepseek-math-7b-instruct\",\"choices\":[{\"index\":0,\"delta\":{\"role\":\"assistant\",\"content\":\" $\\\\\"},\"logprobs\":null,\"finish_reason\":null}]}\n\ndata: {\"id\":\"chatcmpl-pdfuqi90oyqot1qp7jergc\",\"object\":\"chat.completion.chunk\",\"created\":1739867078,\"model\":\"deepseek-math-7b-instruct\",\"system_fingerprint\":\"deepseek-math-7b-instruct\",\"choices\":[{\"index\":0,\"delta\":{\"role\":\"assistant\",\"content\":\"sin\"},\"logprobs\":null,\"finish_reason\":null}]}\n\ndata: {\"id\":\"chatcmpl-pdfuqi90oyqot1qp7jergc\",\"object\":\"chat.completion.chunk\",\"created\":1739867078,\"model\":\"deepseek-math-7b-instruct\",\"system_fingerprint\":\"deepseek-math-7b-instruct\",\"choices\":[{\"index\":0,\"delta\":{\"role\":\"assistant\",\"content\":\" x\"},\"logprobs\":null,\"finish_reason\":null}]}\n\ndata: {\"id\":\"chatcmpl-pdfuqi90oyqot1qp7jergc\",\"object\":\"chat.completion.chunk\",\"created\":1739867078,\"model\":\"deepseek-math-7b-instruct\",\"system_fingerprint\":\"deepseek-math-7b-instruct\",\"choices\":[{\"index\":0,\"delta\":{\"role\":\"assistant\",\"content\":\"=-\"},\"logprobs\":null,\"finish_reason\":null}]}\n\ndata: {\"id\":\"chatcmpl-pdfuqi90oyqot1qp7jergc\",\"object\":\"chat.completion.chunk\",\"created\":1739867078,\"model\":\"deepseek-math-7b-instruct\",\"system_fingerprint\":\"deepseek-math-7b-instruct\",\"choices\":[{\"index\":0,\"delta\":{\"role\":\"assistant\",\"content\":\"1\"},\"logprobs\":null,\"finish_reason\":null}]}\n\ndata: {\"id\":\"chatcmpl-pdfuqi90oyqot1qp7jergc\",\"object\":\"chat.completion.chunk\",\"created\":1739867078,\"model\":\"deepseek-math-7b-instruct\",\"system_fingerprint\":\"deepseek-math-7b-instruct\",\"choices\":[{\"index\":0,\"delta\":{\"role\":\"assistant\",\"content\":\"$\"},\"logprobs\":null,\"finish_reason\":null}]}\n\ndata: {\"id\":\"chatcmpl-pdfuqi90oyqot1qp7jergc\",\"object\":\"chat.completion.chunk\",\"created\":1739867078,\"model\":\"deepseek-math-7b-instruct\",\"system_fingerprint\":\"deepseek-math-7b-instruct\",\"choices\":[{\"index\":0,\"delta\":{\"role\":\"assistant\",\"content\":\" or\"},\"logprobs\":null,\"finish_reason\":null}]}\n\ndata: {\"id\":\"chatcmpl-pdfuqi90oyqot1qp7jergc\",\"object\":\"chat.completion.chunk\",\"created\":1739867078,\"model\":\"deepseek-math-7b-instruct\",\"system_fingerprint\":\"deepseek-math-7b-instruct\",\"choices\":[{\"index\":0,\"delta\":{\"role\":\"assistant\",\"content\":\" $\"},\"logprobs\":null,\"finish_reason\":null}]}\n\ndata: {\"id\":\"chatcmpl-pdfuqi90oyqot1qp7jergc\",\"object\":\"chat.completion.chunk\",\"created\":1739867078,\"model\":\"deepseek-math-7b-instruct\",\"system_fingerprint\":\"deepseek-math-7b-instruct\",\"choices\":[{\"index\":0,\"delta\":{\"role\":\"assistant\",\"content\":\" \"},\"logprobs\":null,\"finish_reason\":null}]}\n\ndata: {\"id\":\"chatcmpl-pdfuqi90oyqot1qp7jergc\",\"object\":\"chat.completion.chunk\",\"created\":1739867078,\"model\":\"deepseek-math-7b-instruct\",\"system_fingerprint\":\"deepseek-math-7b-instruct\",\"choices\":[{\"index\":0,\"delta\":{\"role\":\"assistant\",\"content\":\"2\"},\"logprobs\":null,\"finish_reason\":null}]}\n\ndata: {\"id\":\"chatcmpl-pdfuqi90oyqot1qp7jergc\",\"object\":\"chat.completion.chunk\",\"created\":1739867078,\"model\":\"deepseek-math-7b-instruct\",\"system_fingerprint\":\"deepseek-math-7b-instruct\",\"choices\":[{\"index\":0,\"delta\":{\"role\":\"assistant\",\"content\":\" \\\\\"},\"logprobs\":null,\"finish_reason\":null}]}\n\ndata: {\"id\":\"chatcmpl-pdfuqi90oyqot1qp7jergc\",\"object\":\"chat.completion.chunk\",\"created\":1739867078,\"model\":\"deepseek-math-7b-instruct\",\"system_fingerprint\":\"deepseek-math-7b-instruct\",\"choices\":[{\"index\":0,\"delta\":{\"role\":\"assistant\",\"content\":\"sin\"},\"logprobs\":null,\"finish_reason\":null}]}\n\ndata: {\"id\":\"chatcmpl-pdfuqi90oyqot1qp7jergc\",\"object\":\"chat.completion.chunk\",\"created\":1739867078,\"model\":\"deepseek-math-7b-instruct\",\"system_fingerprint\":\"deepseek-math-7b-instruct\",\"choices\":[{\"index\":0,\"delta\":{\"role\":\"assistant\",\"content\":\" x\"},\"logprobs\":null,\"finish_reason\":null}]}\n\ndata: {\"id\":\"chatcmpl-pdfuqi90oyqot1qp7jergc\",\"object\":\"chat.completion.chunk\",\"created\":1739867078,\"model\":\"deepseek-math-7b-instruct\",\"system_fingerprint\":\"deepseek-math-7b-instruct\",\"choices\":[{\"index\":0,\"delta\":{\"role\":\"assistant\",\"content\":\" +\"},\"logprobs\":null,\"finish_reason\":null}]}\n\ndata: {\"id\":\"chatcmpl-pdfuqi90oyqot1qp7jergc\",\"object\":\"chat.completion.chunk\",\"created\":1739867078,\"model\":\"deepseek-math-7b-instruct\",\"system_fingerprint\":\"deepseek-math-7b-instruct\",\"choices\":[{\"index\":0,\"delta\":{\"role\":\"assistant\",\"content\":\"1\"},\"logprobs\":null,\"finish_reason\":null}]}\n\ndata: {\"id\":\"chatcmpl-pdfuqi90oyqot1qp7jergc\",\"object\":\"chat.completion.chunk\",\"created\":1739867078,\"model\":\"deepseek-math-7b-instruct\",\"system_fingerprint\":\"deepseek-math-7b-instruct\",\"choices\":[{\"index\":0,\"delta\":{\"role\":\"assistant\",\"content\":\" =\"},\"logprobs\":null,\"finish_reason\":null}]}\n\ndata: {\"id\":\"chatcmpl-pdfuqi90oyqot1qp7jergc\",\"object\":\"chat.completion.chunk\",\"created\":1739867078,\"model\":\"deepseek-math-7b-instruct\",\"system_fingerprint\":\"deepseek-math-7b-instruct\",\"choices\":[{\"index\":0,\"delta\":{\"role\":\"assistant\",\"content\":\" \"},\"logprobs\":null,\"finish_reason\":null}]}\n\ndata: {\"id\":\"chatcmpl-pdfuqi90oyqot1qp7jergc\",\"object\":\"chat.completion.chunk\",\"created\":1739867078,\"model\":\"deepseek-math-7b-instruct\",\"system_fingerprint\":\"deepseek-math-7b-instruct\",\"choices\":[{\"index\":0,\"delta\":{\"role\":\"assistant\",\"content\":\"0\"},\"logprobs\":null,\"finish_reason\":null}]}\n\ndata: {\"id\":\"chatcmpl-pdfuqi90oyqot1qp7jergc\",\"object\":\"chat.completion.chunk\",\"created\":1739867078,\"model\":\"deepseek-math-7b-instruct\",\"system_fingerprint\":\"deepseek-math-7b-instruct\",\"choices\":[{\"index\":0,\"delta\":{\"role\":\"assistant\",\"content\":\" $.\"},\"logprobs\":null,\"finish_reason\":null}]}\n\ndata: {\"id\":\"chatcmpl-pdfuqi90oyqot1qp7jergc\",\"object\":\"chat.completion.chunk\",\"created\":1739867078,\"model\":\"deepseek-math-7b-instruct\",\"system_fingerprint\":\"deepseek-math-7b-instruct\",\"choices\":[{\"index\":0,\"delta\":{\"role\":\"assistant\",\"content\":\" The\"},\"logprobs\":null,\"finish_reason\":null}]}\n\ndata: {\"id\":\"chatcmpl-pdfuqi90oyqot1qp7jergc\",\"object\":\"chat.completion.chunk\",\"created\":1739867078,\"model\":\"deepseek-math-7b-instruct\",\"system_fingerprint\":\"deepseek-math-7b-instruct\",\"choices\":[{\"index\":0,\"delta\":{\"role\":\"assistant\",\"content\":\" first\"},\"logprobs\":null,\"finish_reason\":null}]}\n\ndata: {\"id\":\"chatcmpl-pdfuqi90oyqot1qp7jergc\",\"object\":\"chat.completion.chunk\",\"created\":1739867078,\"model\":\"deepseek-math-7b-instruct\",\"system_fingerprint\":\"deepseek-math-7b-instruct\",\"choices\":[{\"index\":0,\"delta\":{\"role\":\"assistant\",\"content\":\" equation\"},\"logprobs\":null,\"finish_reason\":null}]}\n\ndata: {\"id\":\"chatcmpl-pdfuqi90oyqot1qp7jergc\",\"object\":\"chat.completion.chunk\",\"created\":1739867078,\"model\":\"deepseek-math-7b-instruct\",\"system_fingerprint\":\"deepseek-math-7b-instruct\",\"choices\":[{\"index\":0,\"delta\":{\"role\":\"assistant\",\"content\":\" has\"},\"logprobs\":null,\"finish_reason\":null}]}\n\ndata: {\"id\":\"chatcmpl-pdfuqi90oyqot1qp7jergc\",\"object\":\"chat.completion.chunk\",\"created\":1739867078,\"model\":\"deepseek-math-7b-instruct\",\"system_fingerprint\":\"deepseek-math-7b-instruct\",\"choices\":[{\"index\":0,\"delta\":{\"role\":\"assistant\",\"content\":\" the\"},\"logprobs\":null,\"finish_reason\":null}]}\n\ndata: {\"id\":\"chatcmpl-pdfuqi90oyqot1qp7jergc\",\"object\":\"chat.completion.chunk\",\"created\":1739867078,\"model\":\"deepseek-math-7b-instruct\",\"system_fingerprint\":\"deepseek-math-7b-instruct\",\"choices\":[{\"index\":0,\"delta\":{\"role\":\"assistant\",\"content\":\" solutions\"},\"logprobs\":null,\"finish_reason\":null}]}\n\ndata: {\"id\":\"chatcmpl-pdfuqi90oyqot1qp7jergc\",\"object\":\"chat.completion.chunk\",\"created\":1739867078,\"model\":\"deepseek-math-7b-instruct\",\"system_fingerprint\":\"deepseek-math-7b-instruct\",\"choices\":[{\"index\":0,\"delta\":{\"role\":\"assistant\",\"content\":\" of\"},\"logprobs\":null,\"finish_reason\":null}]}\n\ndata: {\"id\":\"chatcmpl-pdfuqi90oyqot1qp7jergc\",\"object\":\"chat.completion.chunk\",\"created\":1739867078,\"model\":\"deepseek-math-7b-instruct\",\"system_fingerprint\":\"deepseek-math-7b-instruct\",\"choices\":[{\"index\":0,\"delta\":{\"role\":\"assistant\",\"content\":\" form\"},\"logprobs\":null,\"finish_reason\":null}]}\n\ndata: {\"id\":\"chatcmpl-pdfuqi90oyqot1qp7jergc\",\"object\":\"chat.completion.chunk\",\"created\":1739867078,\"model\":\"deepseek-math-7b-instruct\",\"system_fingerprint\":\"deepseek-math-7b-instruct\",\"choices\":[{\"index\":0,\"delta\":{\"role\":\"assistant\",\"content\":\" \\\\[\"},\"logprobs\":null,\"finish_reason\":null}]}\n\ndata: {\"id\":\"chatcmpl-pdfuqi90oyqot1qp7jergc\",\"object\":\"chat.completion.chunk\",\"created\":1739867078,\"model\":\"deepseek-math-7b-instruct\",\"system_fingerprint\":\"deepseek-math-7b-instruct\",\"choices\":[{\"index\":0,\"delta\":{\"role\":\"assistant\",\"content\":\"x\"},\"logprobs\":null,\"finish_reason\":null}]}\n\ndata: {\"id\":\"chatcmpl-pdfuqi90oyqot1qp7jergc\",\"object\":\"chat.completion.chunk\",\"created\":1739867078,\"model\":\"deepseek-math-7b-instruct\",\"system_fingerprint\":\"deepseek-math-7b-instruct\",\"choices\":[{\"index\":0,\"delta\":{\"role\":\"assistant\",\"content\":\"=\"},\"logprobs\":null,\"finish_reason\":null}]}\n\ndata: {\"id\":\"chatcmpl-pdfuqi90oyqot1qp7jergc\",\"object\":\"chat.completion.chunk\",\"created\":1739867078,\"model\":\"deepseek-math-7b-instruct\",\"system_fingerprint\":\"deepseek-math-7b-instruct\",\"choices\":[{\"index\":0,\"delta\":{\"role\":\"assistant\",\"content\":\"k\"},\"logprobs\":null,\"finish_reason\":null}]}\n\ndata: {\"id\":\"chatcmpl-pdfuqi90oyqot1qp7jergc\",\"object\":\"chat.completion.chunk\",\"created\":1739867078,\"model\":\"deepseek-math-7b-instruct\",\"system_fingerprint\":\"deepseek-math-7b-instruct\",\"choices\":[{\"index\":0,\"delta\":{\"role\":\"assistant\",\"content\":\"\\\\\"},\"logprobs\":null,\"finish_reason\":null}]}\n\ndata: {\"id\":\"chatcmpl-pdfuqi90oyqot1qp7jergc\",\"object\":\"chat.completion.chunk\",\"created\":1739867078,\"model\":\"deepseek-math-7b-instruct\",\"system_fingerprint\":\"deepseek-math-7b-instruct\",\"choices\":[{\"index\":0,\"delta\":{\"role\":\"assistant\",\"content\":\"pi\"},\"logprobs\":null,\"finish_reason\":null}]}\n\ndata: {\"id\":\"chatcmpl-pdfuqi90oyqot1qp7jergc\",\"object\":\"chat.completion.chunk\",\"created\":1739867078,\"model\":\"deepseek-math-7b-instruct\",\"system_fingerprint\":\"deepseek-math-7b-instruct\",\"choices\":[{\"index\":0,\"delta\":{\"role\":\"assistant\",\"content\":\"-\\\\\"},\"logprobs\":null,\"finish_reason\":null}]}\n\ndata: {\"id\":\"chatcmpl-pdfuqi90oyqot1qp7jergc\",\"object\":\"chat.completion.chunk\",\"created\":1739867078,\"model\":\"deepseek-math-7b-instruct\",\"system_fingerprint\":\"deepseek-math-7b-instruct\",\"choices\":[{\"index\":0,\"delta\":{\"role\":\"assistant\",\"content\":\"frac\"},\"logprobs\":null,\"finish_reason\":null}]}\n\ndata: {\"id\":\"chatcmpl-pdfuqi90oyqot1qp7jergc\",\"object\":\"chat.completion.chunk\",\"created\":1739867078,\"model\":\"deepseek-math-7b-instruct\",\"system_fingerprint\":\"deepseek-math-7b-instruct\",\"choices\":[{\"index\":0,\"delta\":{\"role\":\"assistant\",\"content\":\"{\\\\\"},\"logprobs\":null,\"finish_reason\":null}]}\n\ndata: {\"id\":\"chatcmpl-pdfuqi90oyqot1qp7jergc\",\"object\":\"chat.completion.chunk\",\"created\":1739867078,\"model\":\"deepseek-math-7b-instruct\",\"system_fingerprint\":\"deepseek-math-7b-instruct\",\"choices\":[{\"index\":0,\"delta\":{\"role\":\"assistant\",\"content\":\"pi\"},\"logprobs\":null,\"finish_reason\":null}]}\n\ndata: {\"id\":\"chatcmpl-pdfuqi90oyqot1qp7jergc\",\"object\":\"chat.completion.chunk\",\"created\":1739867078,\"model\":\"deepseek-math-7b-instruct\",\"system_fingerprint\":\"deepseek-math-7b-instruct\",\"choices\":[{\"index\":0,\"delta\":{\"role\":\"assistant\",\"content\":\"}{\"},\"logprobs\":null,\"finish_reason\":null}]}\n\ndata: {\"id\":\"chatcmpl-pdfuqi90oyqot1qp7jergc\",\"object\":\"chat.completion.chunk\",\"created\":1739867078,\"model\":\"deepseek-math-7b-instruct\",\"system_fingerprint\":\"deepseek-math-7b-instruct\",\"choices\":[{\"index\":0,\"delta\":{\"role\":\"assistant\",\"content\":\"2\"},\"logprobs\":null,\"finish_reason\":null}]}\n\ndata: {\"id\":\"chatcmpl-pdfuqi90oyqot1qp7jergc\",\"object\":\"chat.completion.chunk\",\"created\":1739867078,\"model\":\"deepseek-math-7b-instruct\",\"system_fingerprint\":\"deepseek-math-7b-instruct\",\"choices\":[{\"index\":0,\"delta\":{\"role\":\"assistant\",\"content\":\"},\\\\\"},\"logprobs\":null,\"finish_reason\":null}]}\n\ndata: {\"id\":\"chatcmpl-pdfuqi90oyqot1qp7jergc\",\"object\":\"chat.completion.chunk\",\"created\":1739867078,\"model\":\"deepseek-math-7b-instruct\",\"system_fingerprint\":\"deepseek-math-7b-instruct\",\"choices\":[{\"index\":0,\"delta\":{\"role\":\"assistant\",\"content\":\"quad\"},\"logprobs\":null,\"finish_reason\":null}]}\n\ndata: {\"id\":\"chatcmpl-pdfuqi90oyqot1qp7jergc\",\"object\":\"chat.completion.chunk\",\"created\":1739867078,\"model\":\"deepseek-math-7b-instruct\",\"system_fingerprint\":\"deepseek-math-7b-instruct\",\"choices\":[{\"index\":0,\"delta\":{\"role\":\"assistant\",\"content\":\" k\"},\"logprobs\":null,\"finish_reason\":null}]}\n\ndata: {\"id\":\"chatcmpl-pdfuqi90oyqot1qp7jergc\",\"object\":\"chat.completion.chunk\",\"created\":1739867078,\"model\":\"deepseek-math-7b-instruct\",\"system_fingerprint\":\"deepseek-math-7b-instruct\",\"choices\":[{\"index\":0,\"delta\":{\"role\":\"assistant\",\"content\":\"=\\\\\"},\"logprobs\":null,\"finish_reason\":null}]}\n\ndata: {\"id\":\"chatcmpl-pdfuqi90oyqot1qp7jergc\",\"object\":\"chat.completion.chunk\",\"created\":1739867078,\"model\":\"deepseek-math-7b-instruct\",\"system_fingerprint\":\"deepseek-math-7b-instruct\",\"choices\":[{\"index\":0,\"delta\":{\"role\":\"assistant\",\"content\":\"pm\"},\"logprobs\":null,\"finish_reason\":null}]}\n\ndata: {\"id\":\"chatcmpl-pdfuqi90oyqot1qp7jergc\",\"object\":\"chat.completion.chunk\",\"created\":1739867078,\"model\":\"deepseek-math-7b-instruct\",\"system_fingerprint\":\"deepseek-math-7b-instruct\",\"choices\":[{\"index\":0,\"delta\":{\"role\":\"assistant\",\"content\":\"1\"},\"logprobs\":null,\"finish_reason\":null}]}\n\ndata: {\"id\":\"chatcmpl-pdfuqi90oyqot1qp7jergc\",\"object\":\"chat.completion.chunk\",\"created\":1739867078,\"model\":\"deepseek-math-7b-instruct\",\"system_fingerprint\":\"deepseek-math-7b-instruct\",\"choices\":[{\"index\":0,\"delta\":{\"role\":\"assistant\",\"content\":\",\\\\\"},\"logprobs\":null,\"finish_reason\":null}]}\n\ndata: {\"id\":\"chatcmpl-pdfuqi90oyqot1qp7jergc\",\"object\":\"chat.completion.chunk\",\"created\":1739867078,\"model\":\"deepseek-math-7b-instruct\",\"system_fingerprint\":\"deepseek-math-7b-instruct\",\"choices\":[{\"index\":0,\"delta\":{\"role\":\"assistant\",\"content\":\"pm\"},\"logprobs\":null,\"finish_reason\":null}]}\n\ndata: {\"id\":\"chatcmpl-pdfuqi90oyqot1qp7jergc\",\"object\":\"chat.completion.chunk\",\"created\":1739867078,\"model\":\"deepseek-math-7b-instruct\",\"system_fingerprint\":\"deepseek-math-7b-instruct\",\"choices\":[{\"index\":0,\"delta\":{\"role\":\"assistant\",\"content\":\"2\"},\"logprobs\":null,\"finish_reason\":null}]}\n\ndata: {\"id\":\"chatcmpl-pdfuqi90oyqot1qp7jergc\",\"object\":\"chat.completion.chunk\",\"created\":1739867078,\"model\":\"deepseek-math-7b-instruct\",\"system_fingerprint\":\"deepseek-math-7b-instruct\",\"choices\":[{\"index\":0,\"delta\":{\"role\":\"assistant\",\"content\":\",\"},\"logprobs\":null,\"finish_reason\":null}]}\n\ndata: {\"id\":\"chatcmpl-pdfuqi90oyqot1qp7jergc\",\"object\":\"chat.completion.chunk\",\"created\":1739867078,\"model\":\"deepseek-math-7b-instruct\",\"system_fingerprint\":\"deepseek-math-7b-instruct\",\"choices\":[{\"index\":0,\"delta\":{\"role\":\"assistant\",\"content\":\"....\"},\"logprobs\":null,\"finish_reason\":null}]}\n\ndata: {\"id\":\"chatcmpl-pdfuqi90oyqot1qp7jergc\",\"object\":\"chat.completion.chunk\",\"created\":1739867078,\"model\":\"deepseek-math-7b-instruct\",\"system_fingerprint\":\"deepseek-math-7b-instruct\",\"choices\":[{\"index\":0,\"delta\":{\"role\":\"assistant\",\"content\":\"\\\\]\"},\"logprobs\":null,\"finish_reason\":null}]}\n\ndata: {\"id\":\"chatcmpl-pdfuqi90oyqot1qp7jergc\",\"object\":\"chat.completion.chunk\",\"created\":1739867078,\"model\":\"deepseek-math-7b-instruct\",\"system_fingerprint\":\"deepseek-math-7b-instruct\",\"choices\":[{\"index\":0,\"delta\":{\"role\":\"assistant\",\"content\":\"The\"},\"logprobs\":null,\"finish_reason\":null}]}\n\ndata: {\"id\":\"chatcmpl-pdfuqi90oyqot1qp7jergc\",\"object\":\"chat.completion.chunk\",\"created\":1739867078,\"model\":\"deepseek-math-7b-instruct\",\"system_fingerprint\":\"deepseek-math-7b-instruct\",\"choices\":[{\"index\":0,\"delta\":{\"role\":\"assistant\",\"content\":\" second\"},\"logprobs\":null,\"finish_reason\":null}]}\n\ndata: {\"id\":\"chatcmpl-pdfuqi90oyqot1qp7jergc\",\"object\":\"chat.completion.chunk\",\"created\":1739867078,\"model\":\"deepseek-math-7b-instruct\",\"system_fingerprint\":\"deepseek-math-7b-instruct\",\"choices\":[{\"index\":0,\"delta\":{\"role\":\"assistant\",\"content\":\" one\"},\"logprobs\":null,\"finish_reason\":null}]}\n\ndata: {\"id\":\"chatcmpl-pdfuqi90oyqot1qp7jergc\",\"object\":\"chat.completion.chunk\",\"created\":1739867078,\"model\":\"deepseek-math-7b-instruct\",\"system_fingerprint\":\"deepseek-math-7b-instruct\",\"choices\":[{\"index\":0,\"delta\":{\"role\":\"assistant\",\"content\":\" gives\"},\"logprobs\":null,\"finish_reason\":null}]}\n\ndata: {\"id\":\"chatcmpl-pdfuqi90oyqot1qp7jergc\",\"object\":\"chat.completion.chunk\",\"created\":1739867078,\"model\":\"deepseek-math-7b-instruct\",\"system_fingerprint\":\"deepseek-math-7b-instruct\",\"choices\":[{\"index\":0,\"delta\":{\"role\":\"assistant\",\"content\":\" us\"},\"logprobs\":null,\"finish_reason\":null}]}\n\ndata: {\"id\":\"chatcmpl-pdfuqi90oyqot1qp7jergc\",\"object\":\"chat.completion.chunk\",\"created\":1739867078,\"model\":\"deepseek-math-7b-instruct\",\"system_fingerprint\":\"deepseek-math-7b-instruct\",\"choices\":[{\"index\":0,\"delta\":{\"role\":\"assistant\",\"content\":\" a\"},\"logprobs\":null,\"finish_reason\":null}]}\n\ndata: {\"id\":\"chatcmpl-pdfuqi90oyqot1qp7jergc\",\"object\":\"chat.completion.chunk\",\"created\":1739867078,\"model\":\"deepseek-math-7b-instruct\",\"system_fingerprint\":\"deepseek-math-7b-instruct\",\"choices\":[{\"index\":0,\"delta\":{\"role\":\"assistant\",\"content\":\" solution\"},\"logprobs\":null,\"finish_reason\":null}]}\n\ndata: {\"id\":\"chatcmpl-pdfuqi90oyqot1qp7jergc\",\"object\":\"chat.completion.chunk\",\"created\":1739867078,\"model\":\"deepseek-math-7b-instruct\",\"system_fingerprint\":\"deepseek-math-7b-instruct\",\"choices\":[{\"index\":0,\"delta\":{\"role\":\"assistant\",\"content\":\" for\"},\"logprobs\":null,\"finish_reason\":null}]}\n\ndata: {\"id\":\"chatcmpl-pdfuqi90oyqot1qp7jergc\",\"object\":\"chat.completion.chunk\",\"created\":1739867078,\"model\":\"deepseek-math-7b-instruct\",\"system_fingerprint\":\"deepseek-math-7b-instruct\",\"choices\":[{\"index\":0,\"delta\":{\"role\":\"assistant\",\"content\":\" all\"},\"logprobs\":null,\"finish_reason\":null}]}\n\ndata: {\"id\":\"chatcmpl-pdfuqi90oyqot1qp7jergc\",\"object\":\"chat.completion.chunk\",\"created\":1739867078,\"model\":\"deepseek-math-7b-instruct\",\"system_fingerprint\":\"deepseek-math-7b-instruct\",\"choices\":[{\"index\":0,\"delta\":{\"role\":\"assistant\",\"content\":\" integer\"},\"logprobs\":null,\"finish_reason\":null}]}\n\ndata: {\"id\":\"chatcmpl-pdfuqi90oyqot1qp7jergc\",\"object\":\"chat.completion.chunk\",\"created\":1739867078,\"model\":\"deepseek-math-7b-instruct\",\"system_fingerprint\":\"deepseek-math-7b-instruct\",\"choices\":[{\"index\":0,\"delta\":{\"role\":\"assistant\",\"content\":\" values\"},\"logprobs\":null,\"finish_reason\":null}]}\n\ndata: {\"id\":\"chatcmpl-pdfuqi90oyqot1qp7jergc\",\"object\":\"chat.completion.chunk\",\"created\":1739867078,\"model\":\"deepseek-math-7b-instruct\",\"system_fingerprint\":\"deepseek-math-7b-instruct\",\"choices\":[{\"index\":0,\"delta\":{\"role\":\"assistant\",\"content\":\".\"},\"logprobs\":null,\"finish_reason\":null}]}\n\ndata: {\"id\":\"chatcmpl-pdfuqi90oyqot1qp7jergc\",\"object\":\"chat.completion.chunk\",\"created\":1739867078,\"model\":\"deepseek-math-7b-instruct\",\"system_fingerprint\":\"deepseek-math-7b-instruct\",\"choices\":[{\"index\":0,\"delta\":{\"role\":\"assistant\",\"content\":\" So\"},\"logprobs\":null,\"finish_reason\":null}]}\n\ndata: {\"id\":\"chatcmpl-pdfuqi90oyqot1qp7jergc\",\"object\":\"chat.completion.chunk\",\"created\":1739867078,\"model\":\"deepseek-math-7b-instruct\",\"system_fingerprint\":\"deepseek-math-7b-instruct\",\"choices\":[{\"index\":0,\"delta\":{\"role\":\"assistant\",\"content\":\" we\"},\"logprobs\":null,\"finish_reason\":null}]}\n\ndata: {\"id\":\"chatcmpl-pdfuqi90oyqot1qp7jergc\",\"object\":\"chat.completion.chunk\",\"created\":1739867078,\"model\":\"deepseek-math-7b-instruct\",\"system_fingerprint\":\"deepseek-math-7b-instruct\",\"choices\":[{\"index\":0,\"delta\":{\"role\":\"assistant\",\"content\":\" have\"},\"logprobs\":null,\"finish_reason\":null}]}\n\ndata: {\"id\":\"chatcmpl-pdfuqi90oyqot1qp7jergc\",\"object\":\"chat.completion.chunk\",\"created\":1739867078,\"model\":\"deepseek-math-7b-instruct\",\"system_fingerprint\":\"deepseek-math-7b-instruct\",\"choices\":[{\"index\":0,\"delta\":{\"role\":\"assistant\",\"content\":\" in\"},\"logprobs\":null,\"finish_reason\":null}]}\n\ndata: {\"id\":\"chatcmpl-pdfuqi90oyqot1qp7jergc\",\"object\":\"chat.completion.chunk\",\"created\":1739867078,\"model\":\"deepseek-math-7b-instruct\",\"system_fingerprint\":\"deepseek-math-7b-instruct\",\"choices\":[{\"index\":0,\"delta\":{\"role\":\"assistant\",\"content\":\" total\"},\"logprobs\":null,\"finish_reason\":null}]}\n\ndata: {\"id\":\"chatcmpl-pdfuqi90oyqot1qp7jergc\",\"object\":\"chat.completion.chunk\",\"created\":1739867078,\"model\":\"deepseek-math-7b-instruct\",\"system_fingerprint\":\"deepseek-math-7b-instruct\",\"choices\":[{\"index\":0,\"delta\":{\"role\":\"assistant\",\"content\":\":\"},\"logprobs\":null,\"finish_reason\":null}]}\n\ndata: {\"id\":\"chatcmpl-pdfuqi90oyqot1qp7jergc\",\"object\":\"chat.completion.chunk\",\"created\":1739867078,\"model\":\"deepseek-math-7b-instruct\",\"system_fingerprint\":\"deepseek-math-7b-instruct\",\"choices\":[{\"index\":0,\"delta\":{\"role\":\"assistant\",\"content\":\"\\\\[\"},\"logprobs\":null,\"finish_reason\":null}]}\n\ndata: {\"id\":\"chatcmpl-pdfuqi90oyqot1qp7jergc\",\"object\":\"chat.completion.chunk\",\"created\":1739867078,\"model\":\"deepseek-math-7b-instruct\",\"system_fingerprint\":\"deepseek-math-7b-instruct\",\"choices\":[{\"index\":0,\"delta\":{\"role\":\"assistant\",\"content\":\"(\"},\"logprobs\":null,\"finish_reason\":null}]}\n\ndata: {\"id\":\"chatcmpl-pdfuqi90oyqot1qp7jergc\",\"object\":\"chat.completion.chunk\",\"created\":1739867078,\"model\":\"deepseek-math-7b-instruct\",\"system_fingerprint\":\"deepseek-math-7b-instruct\",\"choices\":[{\"index\":0,\"delta\":{\"role\":\"assistant\",\"content\":\"4\"},\"logprobs\":null,\"finish_reason\":null}]}\n\ndata: {\"id\":\"chatcmpl-pdfuqi90oyqot1qp7jergc\",\"object\":\"chat.completion.chunk\",\"created\":1739867078,\"model\":\"deepseek-math-7b-instruct\",\"system_fingerprint\":\"deepseek-math-7b-instruct\",\"choices\":[{\"index\":0,\"delta\":{\"role\":\"assistant\",\"content\":\"n\"},\"logprobs\":null,\"finish_reason\":null}]}\n\ndata: {\"id\":\"chatcmpl-pdfuqi90oyqot1qp7jergc\",\"object\":\"chat.completion.chunk\",\"created\":1739867078,\"model\":\"deepseek-math-7b-instruct\",\"system_fingerprint\":\"deepseek-math-7b-instruct\",\"choices\":[{\"index\":0,\"delta\":{\"role\":\"assistant\",\"content\":\"+\"},\"logprobs\":null,\"finish_reason\":null}]}\n\ndata: {\"id\":\"chatcmpl-pdfuqi90oyqot1qp7jergc\",\"object\":\"chat.completion.chunk\",\"created\":1739867078,\"model\":\"deepseek-math-7b-instruct\",\"system_fingerprint\":\"deepseek-math-7b-instruct\",\"choices\":[{\"index\":0,\"delta\":{\"role\":\"assistant\",\"content\":\"3\"},\"logprobs\":null,\"finish_reason\":null}]}\n\ndata: {\"id\":\"chatcmpl-pdfuqi90oyqot1qp7jergc\",\"object\":\"chat.completion.chunk\",\"created\":1739867078,\"model\":\"deepseek-math-7b-instruct\",\"system_fingerprint\":\"deepseek-math-7b-instruct\",\"choices\":[{\"index\":0,\"delta\":{\"role\":\"assistant\",\"content\":\")\\\\\"},\"logprobs\":null,\"finish_reason\":null}]}\n\ndata: {\"id\":\"chatcmpl-pdfuqi90oyqot1qp7jergc\",\"object\":\"chat.completion.chunk\",\"created\":1739867078,\"model\":\"deepseek-math-7b-instruct\",\"system_fingerprint\":\"deepseek-math-7b-instruct\",\"choices\":[{\"index\":0,\"delta\":{\"role\":\"assistant\",\"content\":\"dfrac\"},\"logprobs\":null,\"finish_reason\":null}]}\n\ndata: {\"id\":\"chatcmpl-pdfuqi90oyqot1qp7jergc\",\"object\":\"chat.completion.chunk\",\"created\":1739867078,\"model\":\"deepseek-math-7b-instruct\",\"system_fingerprint\":\"deepseek-math-7b-instruct\",\"choices\":[{\"index\":0,\"delta\":{\"role\":\"assistant\",\"content\":\" {\\\\\"},\"logprobs\":null,\"finish_reason\":null}]}\n\ndata: {\"id\":\"chatcmpl-pdfuqi90oyqot1qp7jergc\",\"object\":\"chat.completion.chunk\",\"created\":1739867078,\"model\":\"deepseek-math-7b-instruct\",\"system_fingerprint\":\"deepseek-math-7b-instruct\",\"choices\":[{\"index\":0,\"delta\":{\"role\":\"assistant\",\"content\":\"pi\"},\"logprobs\":null,\"finish_reason\":null}]}\n\ndata: {\"id\":\"chatcmpl-pdfuqi90oyqot1qp7jergc\",\"object\":\"chat.completion.chunk\",\"created\":1739867078,\"model\":\"deepseek-math-7b-instruct\",\"system_fingerprint\":\"deepseek-math-7b-instruct\",\"choices\":[{\"index\":0,\"delta\":{\"role\":\"assistant\",\"content\":\"}\"},\"logprobs\":null,\"finish_reason\":null}]}\n\ndata: {\"id\":\"chatcmpl-pdfuqi90oyqot1qp7jergc\",\"object\":\"chat.completion.chunk\",\"created\":1739867078,\"model\":\"deepseek-math-7b-instruct\",\"system_fingerprint\":\"deepseek-math-7b-instruct\",\"choices\":[{\"index\":0,\"delta\":{\"role\":\"assistant\",\"content\":\" {\"},\"logprobs\":null,\"finish_reason\":null}]}\n\ndata: {\"id\":\"chatcmpl-pdfuqi90oyqot1qp7jergc\",\"object\":\"chat.completion.chunk\",\"created\":1739867078,\"model\":\"deepseek-math-7b-instruct\",\"system_fingerprint\":\"deepseek-math-7b-instruct\",\"choices\":[{\"index\":0,\"delta\":{\"role\":\"assistant\",\"content\":\"6\"},\"logprobs\":null,\"finish_reason\":null}]}\n\ndata: {\"id\":\"chatcmpl-pdfuqi90oyqot1qp7jergc\",\"object\":\"chat.completion.chunk\",\"created\":1739867078,\"model\":\"deepseek-math-7b-instruct\",\"system_fingerprint\":\"deepseek-math-7b-instruct\",\"choices\":[{\"index\":0,\"delta\":{\"role\":\"assistant\",\"content\":\"},\"},\"logprobs\":null,\"finish_reason\":null}]}\n\ndata: {\"id\":\"chatcmpl-pdfuqi90oyqot1qp7jergc\",\"object\":\"chat.completion.chunk\",\"created\":1739867078,\"model\":\"deepseek-math-7b-instruct\",\"system_fingerprint\":\"deepseek-math-7b-instruct\",\"choices\":[{\"index\":0,\"delta\":{\"role\":\"assistant\",\"content\":\" (\"},\"logprobs\":null,\"finish_reason\":null}]}\n\ndata: {\"id\":\"chatcmpl-pdfuqi90oyqot1qp7jergc\",\"object\":\"chat.completion.chunk\",\"created\":1739867078,\"model\":\"deepseek-math-7b-instruct\",\"system_fingerprint\":\"deepseek-math-7b-instruct\",\"choices\":[{\"index\":0,\"delta\":{\"role\":\"assistant\",\"content\":\"4\"},\"logprobs\":null,\"finish_reason\":null}]}\n\ndata: {\"id\":\"chatcmpl-pdfuqi90oyqot1qp7jergc\",\"object\":\"chat.completion.chunk\",\"created\":1739867078,\"model\":\"deepseek-math-7b-instruct\",\"system_fingerprint\":\"deepseek-math-7b-instruct\",\"choices\":[{\"index\":0,\"delta\":{\"role\":\"assistant\",\"content\":\"m\"},\"logprobs\":null,\"finish_reason\":null}]}\n\ndata: {\"id\":\"chatcmpl-pdfuqi90oyqot1qp7jergc\",\"object\":\"chat.completion.chunk\",\"created\":1739867078,\"model\":\"deepseek-math-7b-instruct\",\"system_fingerprint\":\"deepseek-math-7b-instruct\",\"choices\":[{\"index\":0,\"delta\":{\"role\":\"assistant\",\"content\":\" -\"},\"logprobs\":null,\"finish_reason\":null}]}\n\ndata: {\"id\":\"chatcmpl-pdfuqi90oyqot1qp7jergc\",\"object\":\"chat.completion.chunk\",\"created\":1739867078,\"model\":\"deepseek-math-7b-instruct\",\"system_fingerprint\":\"deepseek-math-7b-instruct\",\"choices\":[{\"index\":0,\"delta\":{\"role\":\"assistant\",\"content\":\" \"},\"logprobs\":null,\"finish_reason\":null}]}\n\ndata: {\"id\":\"chatcmpl-pdfuqi90oyqot1qp7jergc\",\"object\":\"chat.completion.chunk\",\"created\":1739867078,\"model\":\"deepseek-math-7b-instruct\",\"system_fingerprint\":\"deepseek-math-7b-instruct\",\"choices\":[{\"index\":0,\"delta\":{\"role\":\"assistant\",\"content\":\"1\"},\"logprobs\":null,\"finish_reason\":null}]}\n\ndata: {\"id\":\"chatcmpl-pdfuqi90oyqot1qp7jergc\",\"object\":\"chat.completion.chunk\",\"created\":1739867078,\"model\":\"deepseek-math-7b-instruct\",\"system_fingerprint\":\"deepseek-math-7b-instruct\",\"choices\":[{\"index\":0,\"delta\":{\"role\":\"assistant\",\"content\":\")\"},\"logprobs\":null,\"finish_reason\":null}]}\n\ndata: {\"id\":\"chatcmpl-pdfuqi90oyqot1qp7jergc\",\"object\":\"chat.completion.chunk\",\"created\":1739867078,\"model\":\"deepseek-math-7b-instruct\",\"system_fingerprint\":\"deepseek-math-7b-instruct\",\"choices\":[{\"index\":0,\"delta\":{\"role\":\"assistant\",\"content\":\" \\\\\"},\"logprobs\":null,\"finish_reason\":null}]}\n\ndata: {\"id\":\"chatcmpl-pdfuqi90oyqot1qp7jergc\",\"object\":\"chat.completion.chunk\",\"created\":1739867078,\"model\":\"deepseek-math-7b-instruct\",\"system_fingerprint\":\"deepseek-math-7b-instruct\",\"choices\":[{\"index\":0,\"delta\":{\"role\":\"assistant\",\"content\":\"dfrac\"},\"logprobs\":null,\"finish_reason\":null}]}\n\ndata: {\"id\":\"chatcmpl-pdfuqi90oyqot1qp7jergc\",\"object\":\"chat.completion.chunk\",\"created\":1739867078,\"model\":\"deepseek-math-7b-instruct\",\"system_fingerprint\":\"deepseek-math-7b-instruct\",\"choices\":[{\"index\":0,\"delta\":{\"role\":\"assistant\",\"content\":\"{\"},\"logprobs\":null,\"finish_reason\":null}]}\n\ndata: {\"id\":\"chatcmpl-pdfuqi90oyqot1qp7jergc\",\"object\":\"chat.completion.chunk\",\"created\":1739867078,\"model\":\"deepseek-math-7b-instruct\",\"system_fingerprint\":\"deepseek-math-7b-instruct\",\"choices\":[{\"index\":0,\"delta\":{\"role\":\"assistant\",\"content\":\" \\\\\"},\"logprobs\":null,\"finish_reason\":null}]}\n\ndata: {\"id\":\"chatcmpl-pdfuqi90oyqot1qp7jergc\",\"object\":\"chat.completion.chunk\",\"created\":1739867078,\"model\":\"deepseek-math-7b-instruct\",\"system_fingerprint\":\"deepseek-math-7b-instruct\",\"choices\":[{\"index\":0,\"delta\":{\"role\":\"assistant\",\"content\":\"pi\"},\"logprobs\":null,\"finish_reason\":null}]}\n\ndata: {\"id\":\"chatcmpl-pdfuqi90oyqot1qp7jergc\",\"object\":\"chat.completion.chunk\",\"created\":1739867078,\"model\":\"deepseek-math-7b-instruct\",\"system_fingerprint\":\"deepseek-math-7b-instruct\",\"choices\":[{\"index\":0,\"delta\":{\"role\":\"assistant\",\"content\":\" }{\"},\"logprobs\":null,\"finish_reason\":null}]}\n\ndata: {\"id\":\"chatcmpl-pdfuqi90oyqot1qp7jergc\",\"object\":\"chat.completion.chunk\",\"created\":1739867078,\"model\":\"deepseek-math-7b-instruct\",\"system_fingerprint\":\"deepseek-math-7b-instruct\",\"choices\":[{\"index\":0,\"delta\":{\"role\":\"assistant\",\"content\":\"2\"},\"logprobs\":null,\"finish_reason\":null}]}\n\ndata: {\"id\":\"chatcmpl-pdfuqi90oyqot1qp7jergc\",\"object\":\"chat.completion.chunk\",\"created\":1739867078,\"model\":\"deepseek-math-7b-instruct\",\"system_fingerprint\":\"deepseek-math-7b-instruct\",\"choices\":[{\"index\":0,\"delta\":{\"role\":\"assistant\",\"content\":\"}\\\\]\"},\"logprobs\":null,\"finish_reason\":null}]}\n\ndata: {\"id\":\"chatcmpl-pdfuqi90oyqot1qp7jergc\",\"object\":\"chat.completion.chunk\",\"created\":1739867078,\"model\":\"deepseek-math-7b-instruct\",\"system_fingerprint\":\"deepseek-math-7b-instruct\",\"choices\":[{\"index\":0,\"delta\":{\"role\":\"assistant\",\"content\":\"where\"},\"logprobs\":null,\"finish_reason\":null}]}\n\ndata: {\"id\":\"chatcmpl-pdfuqi90oyqot1qp7jergc\",\"object\":\"chat.completion.chunk\",\"created\":1739867078,\"model\":\"deepseek-math-7b-instruct\",\"system_fingerprint\":\"deepseek-math-7b-instruct\",\"choices\":[{\"index\":0,\"delta\":{\"role\":\"assistant\",\"content\":\" $\"},\"logprobs\":null,\"finish_reason\":null}]}\n\ndata: {\"id\":\"chatcmpl-pdfuqi90oyqot1qp7jergc\",\"object\":\"chat.completion.chunk\",\"created\":1739867078,\"model\":\"deepseek-math-7b-instruct\",\"system_fingerprint\":\"deepseek-math-7b-instruct\",\"choices\":[{\"index\":0,\"delta\":{\"role\":\"assistant\",\"content\":\" m\"},\"logprobs\":null,\"finish_reason\":null}]}\n\ndata: {\"id\":\"chatcmpl-pdfuqi90oyqot1qp7jergc\",\"object\":\"chat.completion.chunk\",\"created\":1739867078,\"model\":\"deepseek-math-7b-instruct\",\"system_fingerprint\":\"deepseek-math-7b-instruct\",\"choices\":[{\"index\":0,\"delta\":{\"role\":\"assistant\",\"content\":\"$\"},\"logprobs\":null,\"finish_reason\":null}]}\n\ndata: {\"id\":\"chatcmpl-pdfuqi90oyqot1qp7jergc\",\"object\":\"chat.completion.chunk\",\"created\":1739867078,\"model\":\"deepseek-math-7b-instruct\",\"system_fingerprint\":\"deepseek-math-7b-instruct\",\"choices\":[{\"index\":0,\"delta\":{\"role\":\"assistant\",\"content\":\" and\"},\"logprobs\":null,\"finish_reason\":null}]}\n\ndata: {\"id\":\"chatcmpl-pdfuqi90oyqot1qp7jergc\",\"object\":\"chat.completion.chunk\",\"created\":1739867078,\"model\":\"deepseek-math-7b-instruct\",\"system_fingerprint\":\"deepseek-math-7b-instruct\",\"choices\":[{\"index\":0,\"delta\":{\"role\":\"assistant\",\"content\":\" $\\\\\"},\"logprobs\":null,\"finish_reason\":null}]}\n\ndata: {\"id\":\"chatcmpl-pdfuqi90oyqot1qp7jergc\",\"object\":\"chat.completion.chunk\",\"created\":1739867078,\"model\":\"deepseek-math-7b-instruct\",\"system_fingerprint\":\"deepseek-math-7b-instruct\",\"choices\":[{\"index\":0,\"delta\":{\"role\":\"assistant\",\"content\":\"displaystyle\"},\"logprobs\":null,\"finish_reason\":null}]}\n\ndata: {\"id\":\"chatcmpl-pdfuqi90oyqot1qp7jergc\",\"object\":\"chat.completion.chunk\",\"created\":1739867078,\"model\":\"deepseek-math-7b-instruct\",\"system_fingerprint\":\"deepseek-math-7b-instruct\",\"choices\":[{\"index\":0,\"delta\":{\"role\":\"assistant\",\"content\":\" n\"},\"logprobs\":null,\"finish_reason\":null}]}\n\ndata: {\"id\":\"chatcmpl-pdfuqi90oyqot1qp7jergc\",\"object\":\"chat.completion.chunk\",\"created\":1739867078,\"model\":\"deepseek-math-7b-instruct\",\"system_fingerprint\":\"deepseek-math-7b-instruct\",\"choices\":[{\"index\":0,\"delta\":{\"role\":\"assistant\",\"content\":\"$\"},\"logprobs\":null,\"finish_reason\":null}]}\n\ndata: {\"id\":\"chatcmpl-pdfuqi90oyqot1qp7jergc\",\"object\":\"chat.completion.chunk\",\"created\":1739867078,\"model\":\"deepseek-math-7b-instruct\",\"system_fingerprint\":\"deepseek-math-7b-instruct\",\"choices\":[{\"index\":0,\"delta\":{\"role\":\"assistant\",\"content\":\" are\"},\"logprobs\":null,\"finish_reason\":null}]}\n\ndata: {\"id\":\"chatcmpl-pdfuqi90oyqot1qp7jergc\",\"object\":\"chat.completion.chunk\",\"created\":1739867078,\"model\":\"deepseek-math-7b-instruct\",\"system_fingerprint\":\"deepseek-math-7b-instruct\",\"choices\":[{\"index\":0,\"delta\":{\"role\":\"assistant\",\"content\":\" integers\"},\"logprobs\":null,\"finish_reason\":null}]}\n\ndata: {\"id\":\"chatcmpl-pdfuqi90oyqot1qp7jergc\",\"object\":\"chat.completion.chunk\",\"created\":1739867078,\"model\":\"deepseek-math-7b-instruct\",\"system_fingerprint\":\"deepseek-math-7b-instruct\",\"choices\":[{\"index\":0,\"delta\":{\"role\":\"assistant\",\"content\":\" as\"},\"logprobs\":null,\"finish_reason\":null}]}\n\ndata: {\"id\":\"chatcmpl-pdfuqi90oyqot1qp7jergc\",\"object\":\"chat.completion.chunk\",\"created\":1739867078,\"model\":\"deepseek-math-7b-instruct\",\"system_fingerprint\":\"deepseek-math-7b-instruct\",\"choices\":[{\"index\":0,\"delta\":{\"role\":\"assistant\",\"content\":\" solutions\"},\"logprobs\":null,\"finish_reason\":null}]}\n\ndata: {\"id\":\"chatcmpl-pdfuqi90oyqot1qp7jergc\",\"object\":\"chat.completion.chunk\",\"created\":1739867078,\"model\":\"deepseek-math-7b-instruct\",\"system_fingerprint\":\"deepseek-math-7b-instruct\",\"choices\":[{\"index\":0,\"delta\":{\"role\":\"assistant\",\"content\":\" of\"},\"logprobs\":null,\"finish_reason\":null}]}\n\ndata: {\"id\":\"chatcmpl-pdfuqi90oyqot1qp7jergc\",\"object\":\"chat.completion.chunk\",\"created\":1739867078,\"model\":\"deepseek-math-7b-instruct\",\"system_fingerprint\":\"deepseek-math-7b-instruct\",\"choices\":[{\"index\":0,\"delta\":{\"role\":\"assistant\",\"content\":\" the\"},\"logprobs\":null,\"finish_reason\":null}]}\n\ndata: {\"id\":\"chatcmpl-pdfuqi90oyqot1qp7jergc\",\"object\":\"chat.completion.chunk\",\"created\":1739867078,\"model\":\"deepseek-math-7b-instruct\",\"system_fingerprint\":\"deepseek-math-7b-instruct\",\"choices\":[{\"index\":0,\"delta\":{\"role\":\"assistant\",\"content\":\" equation\"},\"logprobs\":null,\"finish_reason\":null}]}\n\ndata: {\"id\":\"chatcmpl-pdfuqi90oyqot1qp7jergc\",\"object\":\"chat.completion.chunk\",\"created\":1739867078,\"model\":\"deepseek-math-7b-instruct\",\"system_fingerprint\":\"deepseek-math-7b-instruct\",\"choices\":[{\"index\":0,\"delta\":{\"role\":\"assistant\",\"content\":\",\"},\"logprobs\":null,\"finish_reason\":null}]}\n\ndata: {\"id\":\"chatcmpl-pdfuqi90oyqot1qp7jergc\",\"object\":\"chat.completion.chunk\",\"created\":1739867078,\"model\":\"deepseek-math-7b-instruct\",\"system_fingerprint\":\"deepseek-math-7b-instruct\",\"choices\":[{\"index\":0,\"delta\":{\"role\":\"assistant\",\"content\":\" which\"},\"logprobs\":null,\"finish_reason\":null}]}\n\ndata: {\"id\":\"chatcmpl-pdfuqi90oyqot1qp7jergc\",\"object\":\"chat.completion.chunk\",\"created\":1739867078,\"model\":\"deepseek-math-7b-instruct\",\"system_fingerprint\":\"deepseek-math-7b-instruct\",\"choices\":[{\"index\":0,\"delta\":{\"role\":\"assistant\",\"content\":\" is\"},\"logprobs\":null,\"finish_reason\":null}]}\n\ndata: {\"id\":\"chatcmpl-pdfuqi90oyqot1qp7jergc\",\"object\":\"chat.completion.chunk\",\"created\":1739867078,\"model\":\"deepseek-math-7b-instruct\",\"system_fingerprint\":\"deepseek-math-7b-instruct\",\"choices\":[{\"index\":0,\"delta\":{\"role\":\"assistant\",\"content\":\" equivalent\"},\"logprobs\":null,\"finish_reason\":null}]}\n\ndata: {\"id\":\"chatcmpl-pdfuqi90oyqot1qp7jergc\",\"object\":\"chat.completion.chunk\",\"created\":1739867078,\"model\":\"deepseek-math-7b-instruct\",\"system_fingerprint\":\"deepseek-math-7b-instruct\",\"choices\":[{\"index\":0,\"delta\":{\"role\":\"assistant\",\"content\":\" to\"},\"logprobs\":null,\"finish_reason\":null}]}\n\ndata: {\"id\":\"chatcmpl-pdfuqi90oyqot1qp7jergc\",\"object\":\"chat.completion.chunk\",\"created\":1739867078,\"model\":\"deepseek-math-7b-instruct\",\"system_fingerprint\":\"deepseek-math-7b-instruct\",\"choices\":[{\"index\":0,\"delta\":{\"role\":\"assistant\",\"content\":\"\\n\"},\"logprobs\":null,\"finish_reason\":null}]}\n\ndata: {\"id\":\"chatcmpl-pdfuqi90oyqot1qp7jergc\",\"object\":\"chat.completion.chunk\",\"created\":1739867078,\"model\":\"deepseek-math-7b-instruct\",\"system_fingerprint\":\"deepseek-math-7b-instruct\",\"choices\":[{\"index\":0,\"delta\":{\"role\":\"assistant\",\"content\":\"\\\\[\\\\\"},\"logprobs\":null,\"finish_reason\":null}]}\n\ndata: {\"id\":\"chatcmpl-pdfuqi90oyqot1qp7jergc\",\"object\":\"chat.completion.chunk\",\"created\":1739867078,\"model\":\"deepseek-math-7b-instruct\",\"system_fingerprint\":\"deepseek-math-7b-instruct\",\"choices\":[{\"index\":0,\"delta\":{\"role\":\"assistant\",\"content\":\"left\"},\"logprobs\":null,\"finish_reason\":null}]}\n\ndata: {\"id\":\"chatcmpl-pdfuqi90oyqot1qp7jergc\",\"object\":\"chat.completion.chunk\",\"created\":1739867078,\"model\":\"deepseek-math-7b-instruct\",\"system_fingerprint\":\"deepseek-math-7b-instruct\",\"choices\":[{\"index\":0,\"delta\":{\"role\":\"assistant\",\"content\":\"\\\\{\"},\"logprobs\":null,\"finish_reason\":null}]}\n\ndata: {\"id\":\"chatcmpl-pdfuqi90oyqot1qp7jergc\",\"object\":\"chat.completion.chunk\",\"created\":1739867078,\"model\":\"deepseek-math-7b-instruct\",\"system_fingerprint\":\"deepseek-math-7b-instruct\",\"choices\":[{\"index\":0,\"delta\":{\"role\":\"assistant\",\"content\":\" x\"},\"logprobs\":null,\"finish_reason\":null}]}\n\ndata: {\"id\":\"chatcmpl-pdfuqi90oyqot1qp7jergc\",\"object\":\"chat.completion.chunk\",\"created\":1739867078,\"model\":\"deepseek-math-7b-instruct\",\"system_fingerprint\":\"deepseek-math-7b-instruct\",\"choices\":[{\"index\":0,\"delta\":{\"role\":\"assistant\",\"content\":\"\\\\\"},\"logprobs\":null,\"finish_reason\":null}]}\n\ndata: {\"id\":\"chatcmpl-pdfuqi90oyqot1qp7jergc\",\"object\":\"chat.completion.chunk\",\"created\":1739867078,\"model\":\"deepseek-math-7b-instruct\",\"system_fingerprint\":\"deepseek-math-7b-instruct\",\"choices\":[{\"index\":0,\"delta\":{\"role\":\"assistant\",\"content\":\"in\"},\"logprobs\":null,\"finish_reason\":null}]}\n\ndata: {\"id\":\"chatcmpl-pdfuqi90oyqot1qp7jergc\",\"object\":\"chat.completion.chunk\",\"created\":1739867078,\"model\":\"deepseek-math-7b-instruct\",\"system_fingerprint\":\"deepseek-math-7b-instruct\",\"choices\":[{\"index\":0,\"delta\":{\"role\":\"assistant\",\"content\":\" R\"},\"logprobs\":null,\"finish_reason\":null}]}\n\ndata: {\"id\":\"chatcmpl-pdfuqi90oyqot1qp7jergc\",\"object\":\"chat.completion.chunk\",\"created\":1739867078,\"model\":\"deepseek-math-7b-instruct\",\"system_fingerprint\":\"deepseek-math-7b-instruct\",\"choices\":[{\"index\":0,\"delta\":{\"role\":\"assistant\",\"content\":\" |\"},\"logprobs\":null,\"finish_reason\":null}]}\n\ndata: {\"id\":\"chatcmpl-pdfuqi90oyqot1qp7jergc\",\"object\":\"chat.completion.chunk\",\"created\":1739867078,\"model\":\"deepseek-math-7b-instruct\",\"system_fingerprint\":\"deepseek-math-7b-instruct\",\"choices\":[{\"index\":0,\"delta\":{\"role\":\"assistant\",\"content\":\"x\"},\"logprobs\":null,\"finish_reason\":null}]}\n\ndata: {\"id\":\"chatcmpl-pdfuqi90oyqot1qp7jergc\",\"object\":\"chat.completion.chunk\",\"created\":1739867078,\"model\":\"deepseek-math-7b-instruct\",\"system_fingerprint\":\"deepseek-math-7b-instruct\",\"choices\":[{\"index\":0,\"delta\":{\"role\":\"assistant\",\"content\":\"=\\\\\"},\"logprobs\":null,\"finish_reason\":null}]}\n\ndata: {\"id\":\"chatcmpl-pdfuqi90oyqot1qp7jergc\",\"object\":\"chat.completion.chunk\",\"created\":1739867078,\"model\":\"deepseek-math-7b-instruct\",\"system_fingerprint\":\"deepseek-math-7b-instruct\",\"choices\":[{\"index\":0,\"delta\":{\"role\":\"assistant\",\"content\":\"frac\"},\"logprobs\":null,\"finish_reason\":null}]}\n\ndata: {\"id\":\"chatcmpl-pdfuqi90oyqot1qp7jergc\",\"object\":\"chat.completion.chunk\",\"created\":1739867078,\"model\":\"deepseek-math-7b-instruct\",\"system_fingerprint\":\"deepseek-math-7b-instruct\",\"choices\":[{\"index\":0,\"delta\":{\"role\":\"assistant\",\"content\":\"{(\"},\"logprobs\":null,\"finish_reason\":null}]}\n\ndata: {\"id\":\"chatcmpl-pdfuqi90oyqot1qp7jergc\",\"object\":\"chat.completion.chunk\",\"created\":1739867078,\"model\":\"deepseek-math-7b-instruct\",\"system_fingerprint\":\"deepseek-math-7b-instruct\",\"choices\":[{\"index\":0,\"delta\":{\"role\":\"assistant\",\"content\":\"4\"},\"logprobs\":null,\"finish_reason\":null}]}\n\ndata: {\"id\":\"chatcmpl-pdfuqi90oyqot1qp7jergc\",\"object\":\"chat.completion.chunk\",\"created\":1739867078,\"model\":\"deepseek-math-7b-instruct\",\"system_fingerprint\":\"deepseek-math-7b-instruct\",\"choices\":[{\"index\":0,\"delta\":{\"role\":\"assistant\",\"content\":\"k\"},\"logprobs\":null,\"finish_reason\":null}]}\n\ndata: {\"id\":\"chatcmpl-pdfuqi90oyqot1qp7jergc\",\"object\":\"chat.completion.chunk\",\"created\":1739867078,\"model\":\"deepseek-math-7b-instruct\",\"system_fingerprint\":\"deepseek-math-7b-instruct\",\"choices\":[{\"index\":0,\"delta\":{\"role\":\"assistant\",\"content\":\"-\"},\"logprobs\":null,\"finish_reason\":null}]}\n\ndata: {\"id\":\"chatcmpl-pdfuqi90oyqot1qp7jergc\",\"object\":\"chat.completion.chunk\",\"created\":1739867078,\"model\":\"deepseek-math-7b-instruct\",\"system_fingerprint\":\"deepseek-math-7b-instruct\",\"choices\":[{\"index\":0,\"delta\":{\"role\":\"assistant\",\"content\":\"1\"},\"logprobs\":null,\"finish_reason\":null}]}\n\ndata: {\"id\":\"chatcmpl-pdfuqi90oyqot1qp7jergc\",\"object\":\"chat.completion.chunk\",\"created\":1739867078,\"model\":\"deepseek-math-7b-instruct\",\"system_fingerprint\":\"deepseek-math-7b-instruct\",\"choices\":[{\"index\":0,\"delta\":{\"role\":\"assistant\",\"content\":\")\\\\\"},\"logprobs\":null,\"finish_reason\":null}]}\n\ndata: {\"id\":\"chatcmpl-pdfuqi90oyqot1qp7jergc\",\"object\":\"chat.completion.chunk\",\"created\":1739867078,\"model\":\"deepseek-math-7b-instruct\",\"system_fingerprint\":\"deepseek-math-7b-instruct\",\"choices\":[{\"index\":0,\"delta\":{\"role\":\"assistant\",\"content\":\"pi\"},\"logprobs\":null,\"finish_reason\":null}]}\n\ndata: {\"id\":\"chatcmpl-pdfuqi90oyqot1qp7jergc\",\"object\":\"chat.completion.chunk\",\"created\":1739867078,\"model\":\"deepseek-math-7b-instruct\",\"system_fingerprint\":\"deepseek-math-7b-instruct\",\"choices\":[{\"index\":0,\"delta\":{\"role\":\"assistant\",\"content\":\"}{\"},\"logprobs\":null,\"finish_reason\":null}]}\n\ndata: {\"id\":\"chatcmpl-pdfuqi90oyqot1qp7jergc\",\"object\":\"chat.completion.chunk\",\"created\":1739867078,\"model\":\"deepseek-math-7b-instruct\",\"system_fingerprint\":\"deepseek-math-7b-instruct\",\"choices\":[{\"index\":0,\"delta\":{\"role\":\"assistant\",\"content\":\"6\"},\"logprobs\":null,\"finish_reason\":null}]}\n\ndata: {\"id\":\"chatcmpl-pdfuqi90oyqot1qp7jergc\",\"object\":\"chat.completion.chunk\",\"created\":1739867078,\"model\":\"deepseek-math-7b-instruct\",\"system_fingerprint\":\"deepseek-math-7b-instruct\",\"choices\":[{\"index\":0,\"delta\":{\"role\":\"assistant\",\"content\":\"}\\\\\"},\"logprobs\":null,\"finish_reason\":null}]}\n\ndata: {\"id\":\"chatcmpl-pdfuqi90oyqot1qp7jergc\",\"object\":\"chat.completion.chunk\",\"created\":1739867078,\"model\":\"deepseek-math-7b-instruct\",\"system_fingerprint\":\"deepseek-math-7b-instruct\",\"choices\":[{\"index\":0,\"delta\":{\"role\":\"assistant\",\"content\":\"right\"},\"logprobs\":null,\"finish_reason\":null}]}\n\ndata: {\"id\":\"chatcmpl-pdfuqi90oyqot1qp7jergc\",\"object\":\"chat.completion.chunk\",\"created\":1739867078,\"model\":\"deepseek-math-7b-instruct\",\"system_fingerprint\":\"deepseek-math-7b-instruct\",\"choices\":[{\"index\":0,\"delta\":{\"role\":\"assistant\",\"content\":\"\\\\}\\\\\"},\"logprobs\":null,\"finish_reason\":null}]}\n\ndata: {\"id\":\"chatcmpl-pdfuqi90oyqot1qp7jergc\",\"object\":\"chat.completion.chunk\",\"created\":1739867078,\"model\":\"deepseek-math-7b-instruct\",\"system_fingerprint\":\"deepseek-math-7b-instruct\",\"choices\":[{\"index\":0,\"delta\":{\"role\":\"assistant\",\"content\":\"bigcup\"},\"logprobs\":null,\"finish_reason\":null}]}\n\ndata: {\"id\":\"chatcmpl-pdfuqi90oyqot1qp7jergc\",\"object\":\"chat.completion.chunk\",\"created\":1739867078,\"model\":\"deepseek-math-7b-instruct\",\"system_fingerprint\":\"deepseek-math-7b-instruct\",\"choices\":[{\"index\":0,\"delta\":{\"role\":\"assistant\",\"content\":\" \\\\{\"},\"logprobs\":null,\"finish_reason\":null}]}\n\ndata: {\"id\":\"chatcmpl-pdfuqi90oyqot1qp7jergc\",\"object\":\"chat.completion.chunk\",\"created\":1739867078,\"model\":\"deepseek-math-7b-instruct\",\"system_fingerprint\":\"deepseek-math-7b-instruct\",\"choices\":[{\"index\":0,\"delta\":{\"role\":\"assistant\",\"content\":\"-\\\\\"},\"logprobs\":null,\"finish_reason\":null}]}\n\ndata: {\"id\":\"chatcmpl-pdfuqi90oyqot1qp7jergc\",\"object\":\"chat.completion.chunk\",\"created\":1739867078,\"model\":\"deepseek-math-7b-instruct\",\"system_fingerprint\":\"deepseek-math-7b-instruct\",\"choices\":[{\"index\":0,\"delta\":{\"role\":\"assistant\",\"content\":\"frac\"},\"logprobs\":null,\"finish_reason\":null}]}\n\ndata: {\"id\":\"chatcmpl-pdfuqi90oyqot1qp7jergc\",\"object\":\"chat.completion.chunk\",\"created\":1739867078,\"model\":\"deepseek-math-7b-instruct\",\"system_fingerprint\":\"deepseek-math-7b-instruct\",\"choices\":[{\"index\":0,\"delta\":{\"role\":\"assistant\",\"content\":\"{\\\\\"},\"logprobs\":null,\"finish_reason\":null}]}\n\ndata: {\"id\":\"chatcmpl-pdfuqi90oyqot1qp7jergc\",\"object\":\"chat.completion.chunk\",\"created\":1739867078,\"model\":\"deepseek-math-7b-instruct\",\"system_fingerprint\":\"deepseek-math-7b-instruct\",\"choices\":[{\"index\":0,\"delta\":{\"role\":\"assistant\",\"content\":\"pi\"},\"logprobs\":null,\"finish_reason\":null}]}\n\ndata: {\"id\":\"chatcmpl-pdfuqi90oyqot1qp7jergc\",\"object\":\"chat.completion.chunk\",\"created\":1739867078,\"model\":\"deepseek-math-7b-instruct\",\"system_fingerprint\":\"deepseek-math-7b-instruct\",\"choices\":[{\"index\":0,\"delta\":{\"role\":\"assistant\",\"content\":\"}\"},\"logprobs\":null,\"finish_reason\":null}]}\n\ndata: {\"id\":\"chatcmpl-pdfuqi90oyqot1qp7jergc\",\"object\":\"chat.completion.chunk\",\"created\":1739867078,\"model\":\"deepseek-math-7b-instruct\",\"system_fingerprint\":\"deepseek-math-7b-instruct\",\"choices\":[{\"index\":0,\"delta\":{\"role\":\"assistant\",\"content\":\" {\"},\"logprobs\":null,\"finish_reason\":null}]}\n\ndata: {\"id\":\"chatcmpl-pdfuqi90oyqot1qp7jergc\",\"object\":\"chat.completion.chunk\",\"created\":1739867078,\"model\":\"deepseek-math-7b-instruct\",\"system_fingerprint\":\"deepseek-math-7b-instruct\",\"choices\":[{\"index\":0,\"delta\":{\"role\":\"assistant\",\"content\":\"2\"},\"logprobs\":null,\"finish_reason\":null}]}\n\ndata: {\"id\":\"chatcmpl-pdfuqi90oyqot1qp7jergc\",\"object\":\"chat.completion.chunk\",\"created\":1739867078,\"model\":\"deepseek-math-7b-instruct\",\"system_fingerprint\":\"deepseek-math-7b-instruct\",\"choices\":[{\"index\":0,\"delta\":{\"role\":\"assistant\",\"content\":\"}+\"},\"logprobs\":null,\"finish_reason\":null}]}\n\ndata: {\"id\":\"chatcmpl-pdfuqi90oyqot1qp7jergc\",\"object\":\"chat.completion.chunk\",\"created\":1739867078,\"model\":\"deepseek-math-7b-instruct\",\"system_fingerprint\":\"deepseek-math-7b-instruct\",\"choices\":[{\"index\":0,\"delta\":{\"role\":\"assistant\",\"content\":\" \"},\"logprobs\":null,\"finish_reason\":null}]}\n\ndata: {\"id\":\"chatcmpl-pdfuqi90oyqot1qp7jergc\",\"object\":\"chat.completion.chunk\",\"created\":1739867078,\"model\":\"deepseek-math-7b-instruct\",\"system_fingerprint\":\"deepseek-math-7b-instruct\",\"choices\":[{\"index\":0,\"delta\":{\"role\":\"assistant\",\"content\":\"2\"},\"logprobs\":null,\"finish_reason\":null}]}\n\ndata: {\"id\":\"chatcmpl-pdfuqi90oyqot1qp7jergc\",\"object\":\"chat.completion.chunk\",\"created\":1739867078,\"model\":\"deepseek-math-7b-instruct\",\"system_fingerprint\":\"deepseek-math-7b-instruct\",\"choices\":[{\"index\":0,\"delta\":{\"role\":\"assistant\",\"content\":\" k\"},\"logprobs\":null,\"finish_reason\":null}]}\n\ndata: {\"id\":\"chatcmpl-pdfuqi90oyqot1qp7jergc\",\"object\":\"chat.completion.chunk\",\"created\":1739867078,\"model\":\"deepseek-math-7b-instruct\",\"system_fingerprint\":\"deepseek-math-7b-instruct\",\"choices\":[{\"index\":0,\"delta\":{\"role\":\"assistant\",\"content\":\" \\\\\"},\"logprobs\":null,\"finish_reason\":null}]}\n\ndata: {\"id\":\"chatcmpl-pdfuqi90oyqot1qp7jergc\",\"object\":\"chat.completion.chunk\",\"created\":1739867078,\"model\":\"deepseek-math-7b-instruct\",\"system_fingerprint\":\"deepseek-math-7b-instruct\",\"choices\":[{\"index\":0,\"delta\":{\"role\":\"assistant\",\"content\":\"pi\"},\"logprobs\":null,\"finish_reason\":null}]}\n\ndata: {\"id\":\"chatcmpl-pdfuqi90oyqot1qp7jergc\",\"object\":\"chat.completion.chunk\",\"created\":1739867078,\"model\":\"deepseek-math-7b-instruct\",\"system_fingerprint\":\"deepseek-math-7b-instruct\",\"choices\":[{\"index\":0,\"delta\":{\"role\":\"assistant\",\"content\":\" ,\"},\"logprobs\":null,\"finish_reason\":null}]}\n\ndata: {\"id\":\"chatcmpl-pdfuqi90oyqot1qp7jergc\",\"object\":\"chat.completion.chunk\",\"created\":1739867078,\"model\":\"deepseek-math-7b-instruct\",\"system_fingerprint\":\"deepseek-math-7b-instruct\",\"choices\":[{\"index\":0,\"delta\":{\"role\":\"assistant\",\"content\":\"+\\\\\"},\"logprobs\":null,\"finish_reason\":null}]}\n\ndata: {\"id\":\"chatcmpl-pdfuqi90oyqot1qp7jergc\",\"object\":\"chat.completion.chunk\",\"created\":1739867078,\"model\":\"deepseek-math-7b-instruct\",\"system_fingerprint\":\"deepseek-math-7b-instruct\",\"choices\":[{\"index\":0,\"delta\":{\"role\":\"assistant\",\"content\":\"frac\"},\"logprobs\":null,\"finish_reason\":null}]}\n\ndata: {\"id\":\"chatcmpl-pdfuqi90oyqot1qp7jergc\",\"object\":\"chat.completion.chunk\",\"created\":1739867078,\"model\":\"deepseek-math-7b-instruct\",\"system_fingerprint\":\"deepseek-math-7b-instruct\",\"choices\":[{\"index\":0,\"delta\":{\"role\":\"assistant\",\"content\":\"{\"},\"logprobs\":null,\"finish_reason\":null}]}\n\ndata: {\"id\":\"chatcmpl-pdfuqi90oyqot1qp7jergc\",\"object\":\"chat.completion.chunk\",\"created\":1739867078,\"model\":\"deepseek-math-7b-instruct\",\"system_fingerprint\":\"deepseek-math-7b-instruct\",\"choices\":[{\"index\":0,\"delta\":{\"role\":\"assistant\",\"content\":\"3\"},\"logprobs\":null,\"finish_reason\":null}]}\n\ndata: {\"id\":\"chatcmpl-pdfuqi90oyqot1qp7jergc\",\"object\":\"chat.completion.chunk\",\"created\":1739867078,\"model\":\"deepseek-math-7b-instruct\",\"system_fingerprint\":\"deepseek-math-7b-instruct\",\"choices\":[{\"index\":0,\"delta\":{\"role\":\"assistant\",\"content\":\"\\\\\"},\"logprobs\":null,\"finish_reason\":null}]}\n\ndata: {\"id\":\"chatcmpl-pdfuqi90oyqot1qp7jergc\",\"object\":\"chat.completion.chunk\",\"created\":1739867078,\"model\":\"deepseek-math-7b-instruct\",\"system_fingerprint\":\"deepseek-math-7b-instruct\",\"choices\":[{\"index\":0,\"delta\":{\"role\":\"assistant\",\"content\":\"pi\"},\"logprobs\":null,\"finish_reason\":null}]}\n\ndata: {\"id\":\"chatcmpl-pdfuqi90oyqot1qp7jergc\",\"object\":\"chat.completion.chunk\",\"created\":1739867078,\"model\":\"deepseek-math-7b-instruct\",\"system_fingerprint\":\"deepseek-math-7b-instruct\",\"choices\":[{\"index\":0,\"delta\":{\"role\":\"assistant\",\"content\":\"}{\"},\"logprobs\":null,\"finish_reason\":null}]}\n\ndata: {\"id\":\"chatcmpl-pdfuqi90oyqot1qp7jergc\",\"object\":\"chat.completion.chunk\",\"created\":1739867078,\"model\":\"deepseek-math-7b-instruct\",\"system_fingerprint\":\"deepseek-math-7b-instruct\",\"choices\":[{\"index\":0,\"delta\":{\"role\":\"assistant\",\"content\":\"2\"},\"logprobs\":null,\"finish_reason\":null}]}\n\ndata: {\"id\":\"chatcmpl-pdfuqi90oyqot1qp7jergc\",\"object\":\"chat.completion.chunk\",\"created\":1739867078,\"model\":\"deepseek-math-7b-instruct\",\"system_fingerprint\":\"deepseek-math-7b-instruct\",\"choices\":[{\"index\":0,\"delta\":{\"role\":\"assistant\",\"content\":\"}\"},\"logprobs\":null,\"finish_reason\":null}]}\n\ndata: {\"id\":\"chatcmpl-pdfuqi90oyqot1qp7jergc\",\"object\":\"chat.completion.chunk\",\"created\":1739867078,\"model\":\"deepseek-math-7b-instruct\",\"system_fingerprint\":\"deepseek-math-7b-instruct\",\"choices\":[{\"index\":0,\"delta\":{\"role\":\"assistant\",\"content\":\" +\"},\"logprobs\":null,\"finish_reason\":null}]}\n\ndata: {\"id\":\"chatcmpl-pdfuqi90oyqot1qp7jergc\",\"object\":\"chat.completion.chunk\",\"created\":1739867078,\"model\":\"deepseek-math-7b-instruct\",\"system_fingerprint\":\"deepseek-math-7b-instruct\",\"choices\":[{\"index\":0,\"delta\":{\"role\":\"assistant\",\"content\":\" \"},\"logprobs\":null,\"finish_reason\":null}]}\n\ndata: {\"id\":\"chatcmpl-pdfuqi90oyqot1qp7jergc\",\"object\":\"chat.completion.chunk\",\"created\":1739867078,\"model\":\"deepseek-math-7b-instruct\",\"system_fingerprint\":\"deepseek-math-7b-instruct\",\"choices\":[{\"index\":0,\"delta\":{\"role\":\"assistant\",\"content\":\"2\"},\"logprobs\":null,\"finish_reason\":null}]}\n\ndata: {\"id\":\"chatcmpl-pdfuqi90oyqot1qp7jergc\",\"object\":\"chat.completion.chunk\",\"created\":1739867078,\"model\":\"deepseek-math-7b-instruct\",\"system_fingerprint\":\"deepseek-math-7b-instruct\",\"choices\":[{\"index\":0,\"delta\":{\"role\":\"assistant\",\"content\":\" m\"},\"logprobs\":null,\"finish_reason\":null}]}\n\ndata: {\"id\":\"chatcmpl-pdfuqi90oyqot1qp7jergc\",\"object\":\"chat.completion.chunk\",\"created\":1739867078,\"model\":\"deepseek-math-7b-instruct\",\"system_fingerprint\":\"deepseek-math-7b-instruct\",\"choices\":[{\"index\":0,\"delta\":{\"role\":\"assistant\",\"content\":\"\\\\\"},\"logprobs\":null,\"finish_reason\":null}]}\n\ndata: {\"id\":\"chatcmpl-pdfuqi90oyqot1qp7jergc\",\"object\":\"chat.completion.chunk\",\"created\":1739867078,\"model\":\"deepseek-math-7b-instruct\",\"system_fingerprint\":\"deepseek-math-7b-instruct\",\"choices\":[{\"index\":0,\"delta\":{\"role\":\"assistant\",\"content\":\"pi\"},\"logprobs\":null,\"finish_reason\":null}]}\n\ndata: {\"id\":\"chatcmpl-pdfuqi90oyqot1qp7jergc\",\"object\":\"chat.completion.chunk\",\"created\":1739867078,\"model\":\"deepseek-math-7b-instruct\",\"system_fingerprint\":\"deepseek-math-7b-instruct\",\"choices\":[{\"index\":0,\"delta\":{\"role\":\"assistant\",\"content\":\" |\\\\\"},\"logprobs\":null,\"finish_reason\":null}]}\n\ndata: {\"id\":\"chatcmpl-pdfuqi90oyqot1qp7jergc\",\"object\":\"chat.completion.chunk\",\"created\":1739867078,\"model\":\"deepseek-math-7b-instruct\",\"system_fingerprint\":\"deepseek-math-7b-instruct\",\"choices\":[{\"index\":0,\"delta\":{\"role\":\"assistant\",\"content\":\";\"},\"logprobs\":null,\"finish_reason\":null}]}\n\ndata: {\"id\":\"chatcmpl-pdfuqi90oyqot1qp7jergc\",\"object\":\"chat.completion.chunk\",\"created\":1739867078,\"model\":\"deepseek-math-7b-instruct\",\"system_fingerprint\":\"deepseek-math-7b-instruct\",\"choices\":[{\"index\":0,\"delta\":{\"role\":\"assistant\",\"content\":\"m\"},\"logprobs\":null,\"finish_reason\":null}]}\n\ndata: {\"id\":\"chatcmpl-pdfuqi90oyqot1qp7jergc\",\"object\":\"chat.completion.chunk\",\"created\":1739867078,\"model\":\"deepseek-math-7b-instruct\",\"system_fingerprint\":\"deepseek-math-7b-instruct\",\"choices\":[{\"index\":0,\"delta\":{\"role\":\"assistant\",\"content\":\",\\\\\"},\"logprobs\":null,\"finish_reason\":null}]}\n\ndata: {\"id\":\"chatcmpl-pdfuqi90oyqot1qp7jergc\",\"object\":\"chat.completion.chunk\",\"created\":1739867078,\"model\":\"deepseek-math-7b-instruct\",\"system_fingerprint\":\"deepseek-math-7b-instruct\",\"choices\":[{\"index\":0,\"delta\":{\"role\":\"assistant\",\"content\":\"text\"},\"logprobs\":null,\"finish_reason\":null}]}\n\ndata: {\"id\":\"chatcmpl-pdfuqi90oyqot1qp7jergc\",\"object\":\"chat.completion.chunk\",\"created\":1739867078,\"model\":\"deepseek-math-7b-instruct\",\"system_fingerprint\":\"deepseek-math-7b-instruct\",\"choices\":[{\"index\":0,\"delta\":{\"role\":\"assistant\",\"content\":\"{\"},\"logprobs\":null,\"finish_reason\":null}]}\n\ndata: {\"id\":\"chatcmpl-pdfuqi90oyqot1qp7jergc\",\"object\":\"chat.completion.chunk\",\"created\":1739867078,\"model\":\"deepseek-math-7b-instruct\",\"system_fingerprint\":\"deepseek-math-7b-instruct\",\"choices\":[{\"index\":0,\"delta\":{\"role\":\"assistant\",\"content\":\"integer\"},\"logprobs\":null,\"finish_reason\":null}]}\n\ndata: {\"id\":\"chatcmpl-pdfuqi90oyqot1qp7jergc\",\"object\":\"chat.completion.chunk\",\"created\":1739867078,\"model\":\"deepseek-math-7b-instruct\",\"system_fingerprint\":\"deepseek-math-7b-instruct\",\"choices\":[{\"index\":0,\"delta\":{\"role\":\"assistant\",\"content\":\"},\"},\"logprobs\":null,\"finish_reason\":null}]}\n\ndata: {\"id\":\"chatcmpl-pdfuqi90oyqot1qp7jergc\",\"object\":\"chat.completion.chunk\",\"created\":1739867078,\"model\":\"deepseek-math-7b-instruct\",\"system_fingerprint\":\"deepseek-math-7b-instruct\",\"choices\":[{\"index\":0,\"delta\":{\"role\":\"assistant\",\"content\":\"k\"},\"logprobs\":null,\"finish_reason\":null}]}\n\ndata: {\"id\":\"chatcmpl-pdfuqi90oyqot1qp7jergc\",\"object\":\"chat.completion.chunk\",\"created\":1739867078,\"model\":\"deepseek-math-7b-instruct\",\"system_fingerprint\":\"deepseek-math-7b-instruct\",\"choices\":[{\"index\":0,\"delta\":{\"role\":\"assistant\",\"content\":\"\\\\}.\"},\"logprobs\":null,\"finish_reason\":null}]}\n\ndata: {\"id\":\"chatcmpl-pdfuqi90oyqot1qp7jergc\",\"object\":\"chat.completion.chunk\",\"created\":1739867078,\"model\":\"deepseek-math-7b-instruct\",\"system_fingerprint\":\"deepseek-math-7b-instruct\",\"choices\":[{\"index\":0,\"delta\":{\"role\":\"assistant\",\"content\":\"\\\\]\"},\"logprobs\":null,\"finish_reason\":null}]}\n\ndata: {\"id\":\"chatcmpl-pdfuqi90oyqot1qp7jergc\",\"object\":\"chat.completion.chunk\",\"created\":1739867078,\"model\":\"deepseek-math-7b-instruct\",\"system_fingerprint\":\"deepseek-math-7b-instruct\",\"choices\":[{\"index\":0,\"delta\":{},\"logprobs\":null,\"finish_reason\":\"stop\"}]}\n\ndata: [DONE]"
  # "{\n  \"id\": \"chatcmpl-k1jxexw5tiq31qq68dtcze\",\n  \"object\": \"chat.completion\",\n  \"created\": 1738826205,\n  \"model\": \"deepseek-r1-distill-qwen-32b\",\n  \"choices\": [\n    {\n      \"index\": 0,\n      \"logprobs\": null,\n      \"finish_reason\": \"stop\",\n      \"message\": {\n        \"role\": \"assistant\",\n        \"content\": \"<think>\\n您好！我是由中国的深度求索（DeepSeek）公司开发的智能助手DeepSeek-R1。如您有任何任何问题，我会尽我所能为您提供帮助。\\n</think>\\n\\n您好！我是由中国的深度求索（DeepSeek）公司开发的智能助手DeepSeek-R1。如您有任何任何问题，我会尽我所能为您提供帮助。\"\n      }\n    }\n  ],\n  \"usage\": {\n    \"prompt_tokens\": 5,\n    \"completion_tokens\": 74,\n    \"total_tokens\": 79\n  },\n  \"system_fingerprint\": \"deepseek-r1-distill-qwen-32b\"\n}"
  n1 = case shown="False" "stream" {
    tunnel: [w8 w31] -> w6
    tunnel: [w15 w42] -> w5
    tunnel: [w7 w32] -> w2
    tunnel: "Response JSON" -> [w14 w40]
    tunnel: [_ w30] -> w1
    frame True {
      w13 = "\n\n"  # Codes Display
      n2 = call <vilib>:"Delimited String to 1D String Array.vi"("delimiter"=w13, "delimited string"=w14) -> ("string array"=w12:string[])  [unwired: 9 in]
      n3 = for {
        tunnel: w12 -> [w18] mode=indexing
        tunnel: [w17] -> w11 mode=indexing
        tunnel: "data:" -> [w16]
        # "remove \"data:\""
        n4 = Search and Replace String(input string=w18, search string=w16) -> (result string=w17:string)  [unwired: 6 in, 3 out]
      }
      n5 = while {
        tunnel: [w28] -> w15
        tunnel: w11 -> [w25] mode=indexing
        tunnel: [w20] -> w8 mode=concatenating
        stop <- w28 stop-if-true
        w24 = T3 {"id"="", "object"="", "created"=0, "model"="", "choices"=[]} ("流式应答类型")
        # "Stop when AI response is complete."
        n6 = call <vilib>:"Unflatten From JSON String.vi"("Type and Defaults"=w24, "JSON String"=w25) -> ("error out"=w26:errorcluster, "Variant"=w27:variant)  [unwired: 8 in]
        n7 = Variant To Data(error in=w26, type=w24, Variant=w27) -> (data=w23:T3)  [unwired: 1 out]
        n8 = Unbundle By Name(w23) -> ("choices"=w22:T4)
        n9 = Index Array(array=w22) -> (element=w21:T5)  [unwired: 1 in]
        n10 = Unbundle By Name(w21) -> ("delta.content"=w20:string, "finish_reason"=w19:string)
        n11 = Equal?(x=w19, y="stop") -> (x = y?=w28:bool)
      }
      n12 = Bundle By Name(cluster=T1 {"role"=enum."assistant", "content"="", "reasoning"=""} ("Data"), "content"=w8) -> (w7:T1)
    }
    frame False {
      w37 = T6 {"id"="", "object"="", "created"=0, "model"="", "choices"=[]} ("Response类型")
      n13 = call <vilib>:"Unflatten From JSON String.vi"("Type and Defaults"=w37, "JSON String"=w40) -> ("error out"=w39:errorcluster, "Variant"=w38:variant)  [unwired: 8 in]
      n14 = Variant To Data(error in=w39, type=w37, Variant=w38) -> (data=w36:T6)  [unwired: 1 out]
      n15 = Unbundle By Name(w36) -> ("choices"=w35:T7)
      n16 = Index Array(array=w35) -> (element=w34:T8)  [unwired: 1 in]
      n17 = Unbundle By Name(w34) -> ("message.reasoning"=w30:string, "message.content"=w31:string, "finish_reason"=w33:string, "message"=w32:T1)
      n18 = Equal?(x=w33, y="stop") -> (x = y?=w42:bool)
    }
  }
  "answer" <- w6
  "complete?" <- w5
  "message" <- w2
  "openrouter reasoning" <- w1
